vi "SCA-RT.vi"() -> ()   [LabVIEW 2016]
uses:
  controls/SCA states.ctl
  Common-Control/Gate Valve Readback.ctl
  controls/Vertical Rod states.ctl
  Common-Control/Horizontal Rod states.ctl
  Common-Control/GP307 cluster.ctl
  controls/SCA commands.ctl
  controls/SCA Bypass control.ctl
  <vilib>/Platform/TimedLoop/XDataNode/timing_clust.ctl
  <vilib>/Platform/TimedLoop/XDataNode/nitl_modes.ctl
  <vilib>/Platform/TimedLoop/XDataNode/wakeup.ctl
  controls/Encoder bit cluster.ctl
  controls/Minimum Times.ctl
  <vilib>/Analysis/baseanly.llb/Mean (DBL).vi
  <vilib>/Instr/_visa.llb/VISA Configure Serial Port (Instr).vi
  <vilib>/Motion/Express/_s/nimc.fb.straightLineMove.startStraightLineMove.axis.modeRelative.0.vi
  <vilib>/Platform/TimedLoop/XDataNode/loadnilvce.vi
  <vilib>/Motion/BlockNode/FB.NIMotion.xnode
  <vilib>/Platform/TimedLoop/XDataNode/XDataNode.xnode
  <vilib>/Platform/TimedLoop/XDataNode/XDNodeRunTimeDep.lvlib
  <vilib>/Analysis/NI_AALBase.lvlib
  <vilib>/NI_Real-Time Target Support.lvlib
panel:
  in  "Insert Rod Bypass":bool
  in  "Retract Rod Bypass":bool
  in  "Sample Rod Bypass":bool
  in  "Wheel GV Bypass":bool
  out "Bypass Control":T1
  out "Timeouts":T2
  out "Immersion Lens I set":dbl
  out "Immersion Lens V Set":dbl
  out "Timeouts Update loop error":errorcluster
  out "SCA Command":T3
  out "Encoder loop error":errorcluster
  out "Convectron readback loop error":errorcluster
  out "HV Control loop error":errorcluster
  out "Rotate Wheel error":errorcluster
  out "Ion Source Vac Cluster":T4
  out "Bellows Vac Cluster":T4
  out "SCA-cRIO error":errorcluster
  in  "Rollover Sample":i8=54
  out "Insert Rod Status":T5
  out "Retract Rod Status":T5
  out "Sample Rod status":T6
  out "Wheel GV":T7
  out "Raw bits":bool[](array[boolean])
  out "Converted bits":bool[](array[boolean])
  out "Immersion Lens I read":dbl format="%0.2f"
  out "Immersion Lens V read":dbl format="%0.2f"
  out "SCA next state":T8
  out "Extractor I read":dbl
  out "Extractor V read":dbl
  out "Extractor V set":dbl
  out "Cathode V read":dbl
  out "Cathode I read":dbl
  out "Cathode V set":dbl
  out "New Move":dbl
  out "Encoder Destination":dbl
  in  "Step Window Radius":i16=2
  out "In Range?":bool
  out "Window Limit 2":u32
  out "Window Limit 1":u32
  out "Encoder position":u16
  in  "clear error 3":bool
  in  "clear error 2":bool
  in  "clear error":bool
  out "action":string
  out "Vac Readback Loop error":errorcluster
  out "Sample Wheel Convectron":string
  out "Sample Rod UP sensor":bool
  out "Sample Rod DOWN sensor":bool
  out "Rotation done":bool
  out "Insert Rod IN sensor":bool
  out "Insert Rod OUT sensor":bool
  out "Retract Rod IN sensor":bool
  out "Retract Rod OUT sensor":bool
  out "Sensor loop error":errorcluster
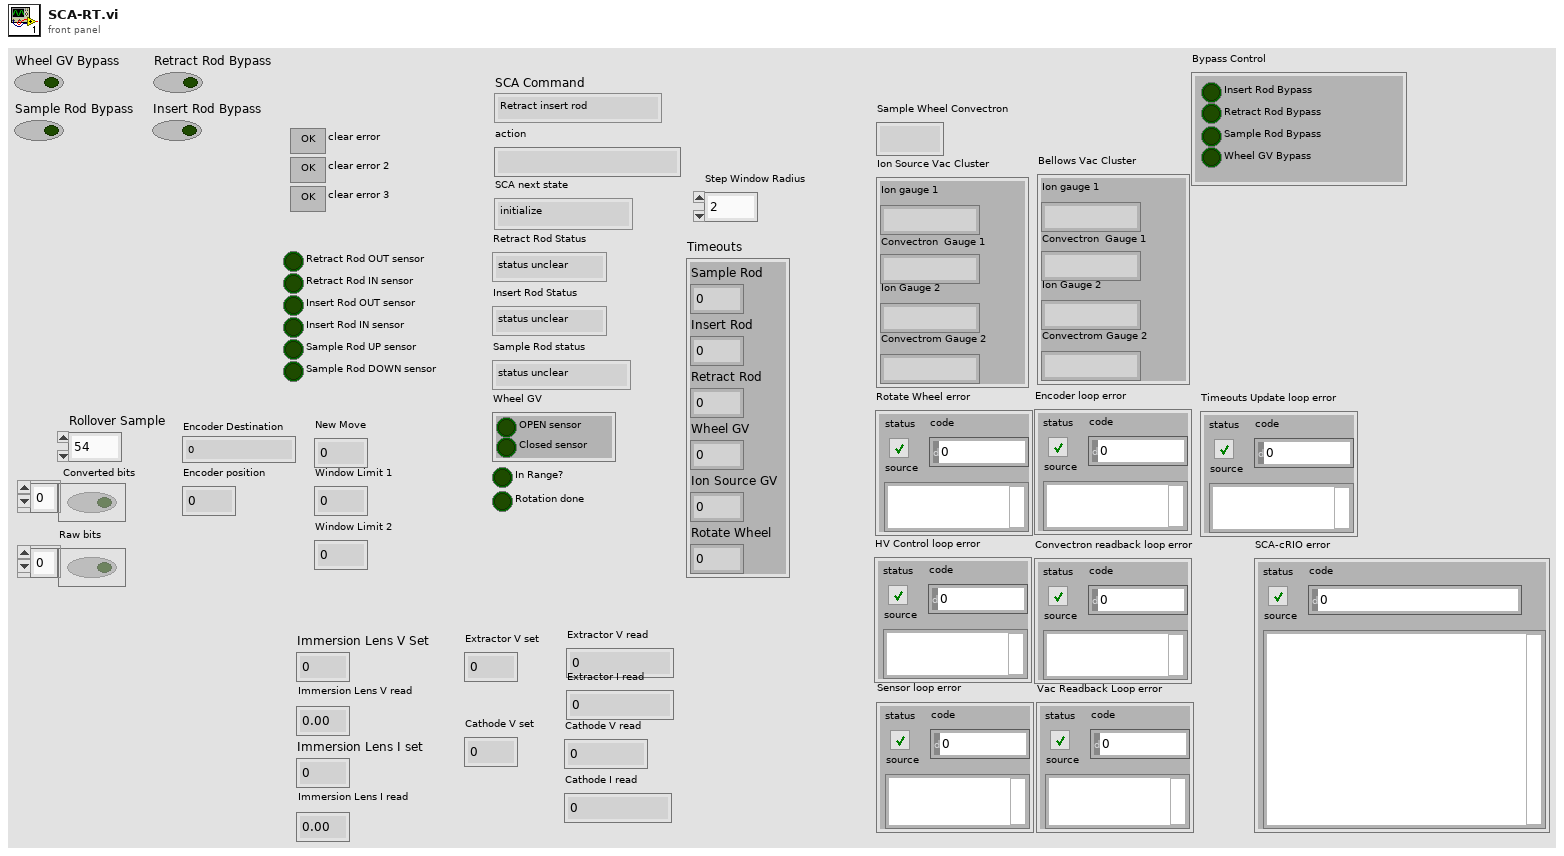
[diagram p1: front panel]
types:
  T1 = typedef "SCA Bypass control.ctl" = cluster{"Insert Rod Bypass":bool, "Retract Rod Bypass":bool, "Sample Rod Bypass":bool, "Wheel GV Bypass":bool}
  T2 = cluster{"Sample Rod":u16, "Insert Rod":u16, "Retract Rod":u16, "Wheel GV":u16, "Ion Source GV":u16, "Rotate Wheel":u16}
  T3 = typedef "SCA commands.ctl" = enum16{"Retract insert rod", "Insert insert rod", "Retract retract rod", "Insert retract rod", "Retract sample rod", "Insert sample rod", "Open wheel GV", "Close wheel GV", "Open ion source GV", "Close ion source GV", "Pump out source", "Vent source", "Rotate wheel randomly", "Rotate wheel", "Start random sample change", "Start sample change"}
  T4 = typedef "GP307 cluster.ctl" = cluster{"Ion gauge 1":string, "Convectron  Gauge 1 ":string, "Ion Gauge 2":string, "Convectrom Gauge 2":string}
  T5 = typedef "Horizontal Rod states.ctl" = enum16{"status unclear", "rod in", "rod out"}
  T6 = typedef "Vertical Rod states.ctl" = enum16{"status unclear", "rod down", "rod up"}
  T7 = typedef "Gate Valve Readback.ctl" = cluster{"OPEN sensor":bool, "Closed sensor":bool}
  T8 = typedef "SCA states.ctl" = enum16{"initialize", "wait", "change sample start", "change sample", "check position", "rotate wheel", "sample change complete", "sample rod up", "sample rod down", "retract rod in", "retract rod out", "insert rod in", "insert rod out", "wheel GV open", "wheel GV close", "vent source", "pump source"}
  T9 = cluster{"Sample Rod":u32, "Insert Rod":u32, "Retract Rod":u32, "Wheel GV":u32, "Ion Source GV":u32, "Rotate Wheel":u32}
  T10 = typedef "Minimum Times.ctl" = cluster{"Rotate Wheel Minimum Time":u32}
  T11 = typedef "GV states.ctl" = enum16{"status unclear", "closed", "open"}
  T12 = typedef "XDNodeRunTimeDep.lvlib/timing_clust.ctl" = cluster{"Expected End [f-1]":u64, "Actual End [f-1]":u64, "Finished Late? [f-1]":bool, "Expected End [i-1]":u64, "Actual End [i-1]":u64, "Finished Late? [i-1]":bool, "Expected Start [i]":u64, "Actual Start [i]":u64, "Expected Start [f]":u64, "Actual Start [f]":u64, "Source Name":string, "Structure Name":string, "Period":i64, "Deadline":i64, "Offset":i64, "Start":i64, "Priority":i32, "Timeout":i32, "Mode":T13, "Wakeup Reason":T14, "Error":errorcluster, "Source Type":string, "Secondary Source Type":string, "Global End Time":u64, "Global Start Time":u64, "Frame Duration":u64, "Iteration Duration":u64, "Assigned CPU":i32, "I/O Scan Engine Mode":u32}
  T13 = typedef "XDNodeRunTimeDep.lvlib/nitl_modes.ctl" = enum32{"No Change", "Process missed periods, maintain original phase", "Discard missed periods, maintain original phase", "Process missed periods, ignore original phase", "Discard missed periods, ignore original phase"}
  T14 = typedef "XDNodeRunTimeDep.lvlib/wakeup.ctl" = enum32{"Normal", "Aborted", "Asynchronous wakeup", "Timing source error", "Timed loop error", "Timeout"}
  T15 = typedef "Encoder bit cluster.ctl" = cluster{"MSB":bool, "13th bit":bool, "12th bit":bool, "11th bit":bool, "10th bit":bool, "9th bit":bool, "8th bit":bool, "7th bit":bool, "6th bit":bool, "5th bit":bool, "4th bit":bool, "3rd bit":bool, "2nd bit":bool, "LSB":bool}
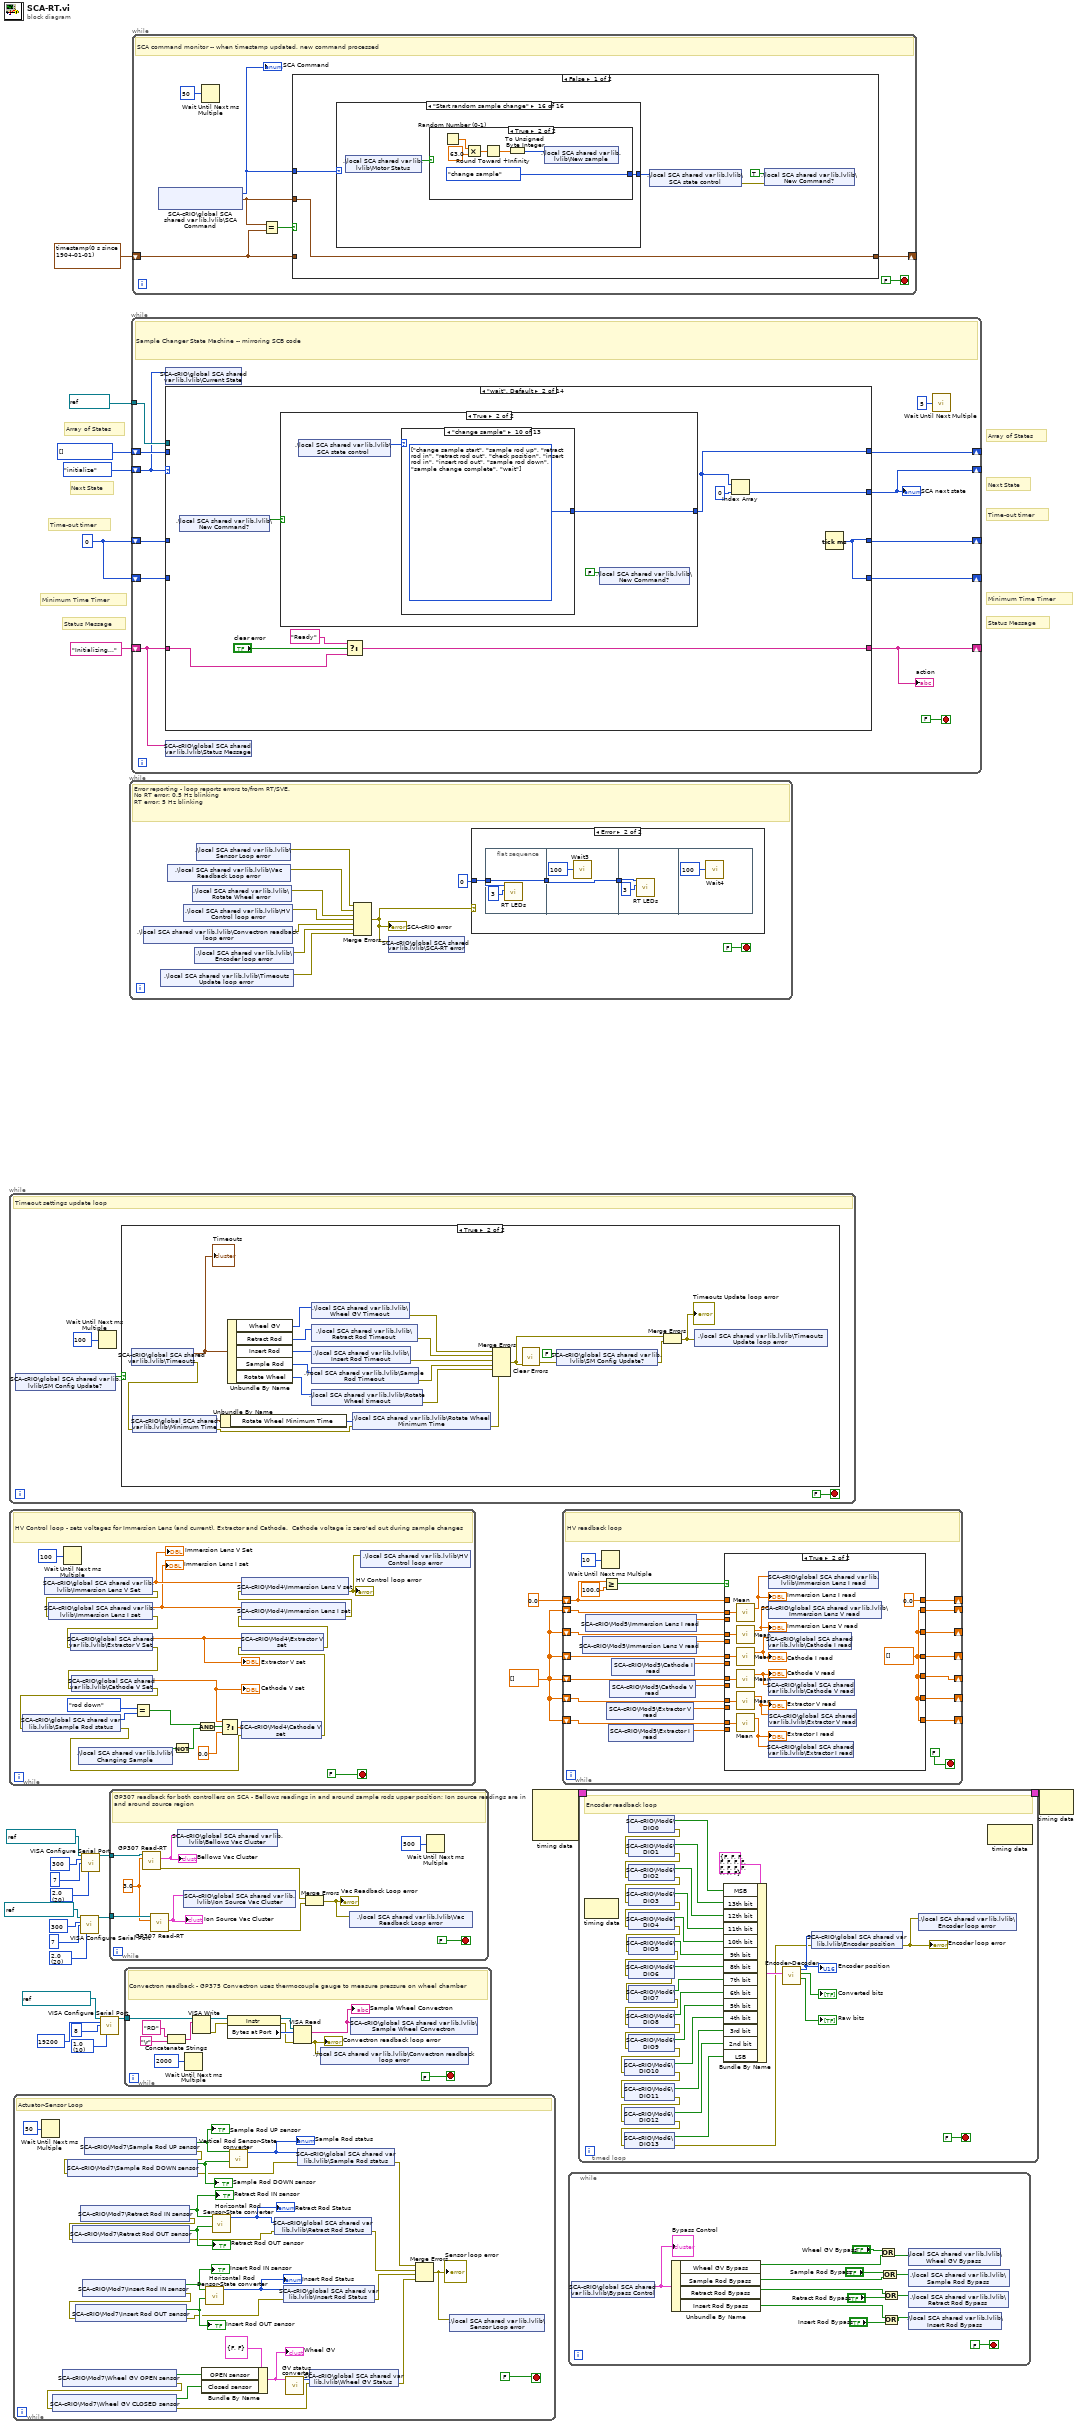
[diagram p0: block diagram]
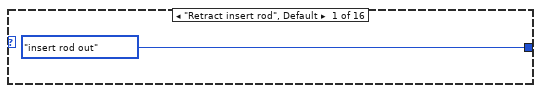
[diagram p2: hidden frame]
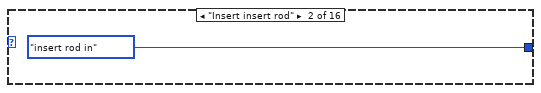
[diagram p3: hidden frame]
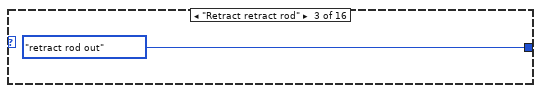
[diagram p4: hidden frame]
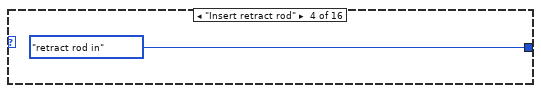
[diagram p5: hidden frame]
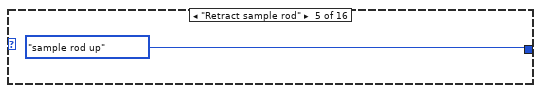
[diagram p6: hidden frame]
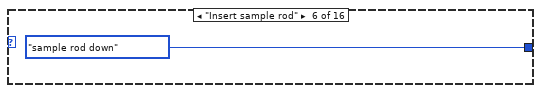
[diagram p7: hidden frame]
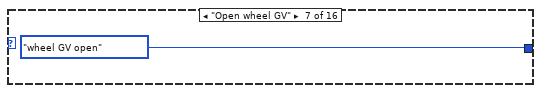
[diagram p8: hidden frame]
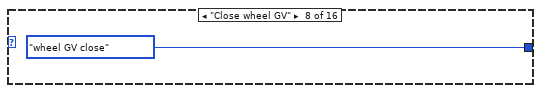
[diagram p9: hidden frame]
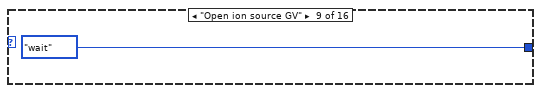
[diagram p10: hidden frame]
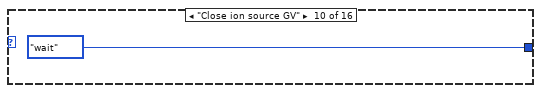
[diagram p11: hidden frame]
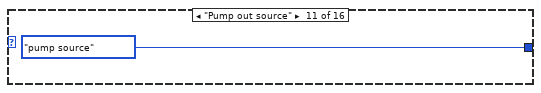
[diagram p12: hidden frame]
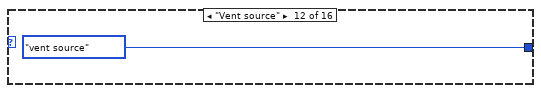
[diagram p13: hidden frame]
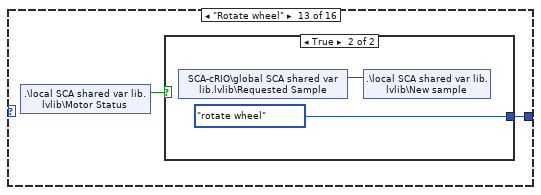
[diagram p14: hidden frame]
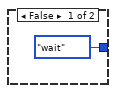
[diagram p15: hidden frame]
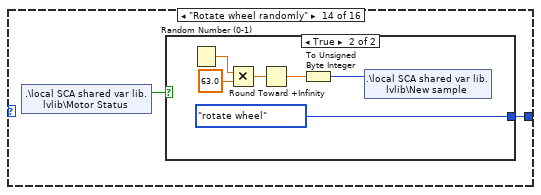
[diagram p16: hidden frame]
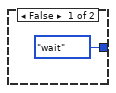
[diagram p17: hidden frame]
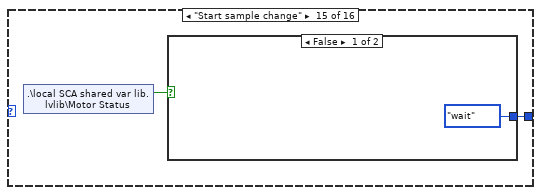
[diagram p18: hidden frame]
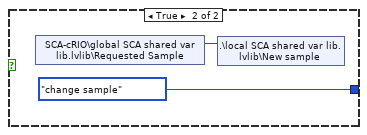
[diagram p19: hidden frame]
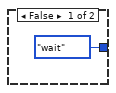
[diagram p20: hidden frame]
diagram:
  w3 = dbl[] []
  w20 = u16 20 items=["1.0"=10, "1.5"=15, "2.0"=20] ("stop bits (10: 1 bit)")
  w24 = u16 10 items=["1.0"=10, "1.5"=15, "2.0"=20] ("stop bits (10: 1 bit)")
  w14 = u16 20 items=["1.0"=10, "1.5"=15, "2.0"=20] ("stop bits (10: 1 bit)")
  w8 = u32 0
  w25 = T8[] [] items=["initialize", "wait", "change sample start", "change sample", "check position", "rotate wheel", "sample change complete", "sample rod up", "sample rod down", "retract rod in", "retract rod out", "insert rod in", "insert rod out", "wheel GV open", "wheel GV close", "vent source", "pump source"]
  # "Status Message"
  # "Array of States"
  # "Next State"
  # "Time-out timer"
  # "Minimum Time Timer"
  # "Status Message"
  # "Array of States"
  # "Next State"
  # "Time-out timer"
  # "Minimum Time Timer"
  n1 = while {
    stop <- FALSE stop-if-true
    # "Timeout settings update loop"
    n2 = shared-variable "SCA-cRIO\\global SCA shared var lib.lvlib\\SM Config Update?"() -> (w28:bool)  [unwired: 1 in, 1 out]
    n3 = Wait Until Next ms Multiple(millisecond multiple=u32 100) -> ()  [unwired: 1 out]
    n4 = case shown="True" w28 {
      frame False {
      }
      frame True {
        n5 = shared-variable "SCA-cRIO\\global SCA shared var lib.lvlib\\Timeouts"() -> (w48:T9, error out=w31:errorcluster)  [unwired: 1 in]
        "Timeouts" <- w48
        n6 = shared-variable "SCA-cRIO\\global SCA shared var lib.lvlib\\Minimum Time"(error in=w31) -> (w33:T10, error out=w30:errorcluster)
        n7 = Unbundle By Name(w33) -> ("Rotate Wheel Minimum Time"=w32:u32)
        n8 = Unbundle By Name(w48) -> ("Wheel GV"=w47:u32, "Retract Rod"=w34:u32, "Insert Rod"=w41:u32, "Sample Rod"=w38:u32, "Rotate Wheel"=w37:u32)
        n9 = shared-variable ".\\local SCA shared var lib.lvlib\\Wheel GV Timeout"(w47) -> (error out=w46:errorcluster)  [unwired: 1 in]
        n10 = shared-variable ".\\local SCA shared var lib.lvlib\\Retract Rod Timeout"(w34) -> (error out=w40:errorcluster)  [unwired: 1 in]
        n11 = shared-variable ".\\local SCA shared var lib.lvlib\\Insert Rod Timeout"(w41) -> (error out=w39:errorcluster)  [unwired: 1 in]
        n12 = shared-variable ".\\local SCA shared var lib.lvlib\\Sample Rod Timeout"(w38) -> (error out=w36:errorcluster)  [unwired: 1 in]
        n13 = shared-variable ".\\local SCA shared var lib.lvlib\\Rotate Wheel timeout"(w37) -> (error out=w35:errorcluster)  [unwired: 1 in]
        n14 = shared-variable ".\\local SCA shared var lib.lvlib\\Rotate Wheel Minimum Time"(w32, error in=w30) -> (error out=w29:errorcluster)
        n15 = Merge Errors(w46, w40, w39, w36, w35, w29) -> (w44:errorcluster)
        n16 = call <vilib>:"Clear Errors.vi"("error in (no error)"=w44) -> ("error out"=w45:errorcluster)  [unwired: 5 in, 1 out]
        n17 = shared-variable "SCA-cRIO\\global SCA shared var lib.lvlib\\SM Config Update?"(FALSE ("SM Config Update?"), error in=w45) -> (error out=w43:errorcluster)
        n18 = Merge Errors(w44, w43) -> (w42:errorcluster)
        "Timeouts Update loop error" <- w42
        n19 = shared-variable ".\\local SCA shared var lib.lvlib\\Timeouts Update loop error"(w42) -> ()  [unwired: 1 in, 1 out]
      }
    }
  }
  n20 = while {
    stop <- FALSE stop-if-true
    # "HV Control loop - sets voltages for Immersion Lens (and current), Extractor and Cathode.  Cathode voltage is zero'ed out during sample changes"
    n21 = shared-variable "SCA-cRIO\\global SCA shared var lib.lvlib\\Immersion Lens V Set"() -> (w64:dbl, error out=w62:errorcluster)  [unwired: 1 in]
    "Immersion Lens V Set" <- w64
    n22 = shared-variable "SCA-cRIO\\global SCA shared var lib.lvlib\\Immersion Lens I set"(error in=w62) -> (w63:dbl, error out=w61:errorcluster)
    "Immersion Lens I set" <- w63
    n23 = Wait Until Next ms Multiple(millisecond multiple=u32 100) -> ()  [unwired: 1 out]
    n24 = shared-variable "SCA-cRIO\\global SCA shared var lib.lvlib\\Extractor V Set"(error in=w61) -> (w70:dbl, error out=w60:errorcluster)
    "Extractor V set" <- w70
    n25 = shared-variable "SCA-cRIO\\global SCA shared var lib.lvlib\\Cathode V Set"(error in=w60) -> (w67:dbl, error out=w59:errorcluster)
    "Cathode V set" <- w67
    n26 = shared-variable "SCA-cRIO\\global SCA shared var lib.lvlib\\Sample Rod status"(error in=w59) -> (w53:T6, error out=w51:errorcluster)
    n27 = shared-variable ".\\local SCA shared var lib.lvlib\\Changing Sample"() -> (w69:bool)  [unwired: 1 in, 1 out]
    n28 = Equal?(x=Vertical_Rod_states."rod down", y=w53) -> (x = y?=w54:bool)
    n29 = Not(x=w69) -> (.not. x?=w50:bool)
    n30 = And(x=w54, y=w50) -> (x .and. y?=w68:bool)
    n31 = Select(t=w67, s=w68, f=0.0) -> (s? t:f=w65:dbl)
    n32 = shared-variable "SCA-cRIO\\Mod4\\Cathode V set"(w65, error in=w51) -> (error out=w56:errorcluster)
    n33 = shared-variable "SCA-cRIO\\Mod4\\Extractor V set"(w70, error in=w56) -> (error out=w57:errorcluster)
    n34 = shared-variable "SCA-cRIO\\Mod4\\Immersion Lens I set"(w63, error in=w57) -> (error out=w58:errorcluster)
    n35 = shared-variable "SCA-cRIO\\Mod4\\Immersion Lens V set"(w64, error in=w58) -> (error out=w55:errorcluster)
    "HV Control loop error" <- w55
    n36 = shared-variable ".\\local SCA shared var lib.lvlib\\HV Control loop error"(w55) -> ()  [unwired: 1 in, 1 out]
  }
  n37 = while {
    stop <- FALSE ("stop") stop-if-true
    # "Actuator-Sensor Loop"
    n38 = Wait Until Next ms Multiple(millisecond multiple=u32 50) -> ()  [unwired: 1 out]
    n39 = shared-variable "SCA-cRIO\\Mod7\\Wheel GV OPEN sensor"() -> (w96:bool, error out=w82:errorcluster)  [unwired: 1 in]
    n40 = shared-variable "SCA-cRIO\\Mod7\\Wheel GV CLOSED sensor"(error in=w82) -> (w97:bool, error out=w81:errorcluster)
    n41 = shared-variable "SCA-cRIO\\Mod7\\Retract Rod IN sensor"() -> (w91:bool, error out=w84:errorcluster)  [unwired: 1 in]
    "Retract Rod IN sensor" <- w91
    n42 = shared-variable "SCA-cRIO\\Mod7\\Retract Rod OUT sensor"(error in=w84) -> (w90:bool, error out=w78:errorcluster)
    "Retract Rod OUT sensor" <- w90
    n43 = shared-variable "SCA-cRIO\\Mod7\\Insert Rod IN sensor"() -> (w89:bool, error out=w83:errorcluster)  [unwired: 1 in]
    "Insert Rod IN sensor" <- w89
    n44 = shared-variable "SCA-cRIO\\Mod7\\Insert Rod OUT sensor"(error in=w83) -> (w88:bool, error out=w80:errorcluster)
    "Insert Rod OUT sensor" <- w88
    n45 = shared-variable "SCA-cRIO\\Mod7\\Sample Rod UP sensor"() -> (w94:bool, error out=w85:errorcluster)  [unwired: 1 in]
    "Sample Rod UP sensor" <- w94
    n46 = shared-variable "SCA-cRIO\\Mod7\\Sample Rod DOWN sensor"(error in=w85) -> (w93:bool, error out=w79:errorcluster)
    "Sample Rod DOWN sensor" <- w93
    n47 = Bundle By Name(cluster=T7 {"OPEN sensor"=FALSE, "Closed sensor"=FALSE} ("Gate Valve"), "OPEN sensor"=w96, "Closed sensor"=w97) -> (w99:T7)
    "Wheel GV" <- w99
    n48 = call "Horizontal Rod Sensor-State converter.vi"("IN Sensor"=w89, "OUT Sensor"=w88) -> ("Status"=w87:T5)  [unwired: 8 in]
    "Insert Rod Status" <- w87
    n49 = call "Horizontal Rod Sensor-State converter.vi"("IN Sensor"=w91, "OUT Sensor"=w90) -> ("Status"=w86:T5)  [unwired: 8 in]
    "Retract Rod Status" <- w86
    n50 = call "Vertical Rod Sensor-State converter.vi"("UP Sensor"=w94, "DOWN Sensor"=w93) -> ("Status"=w92:T6)  [unwired: 8 in]
    "Sample Rod status" <- w92
    n51 = shared-variable "SCA-cRIO\\global SCA shared var lib.lvlib\\Retract Rod Status"(w86, error in=w78) -> (error out=w75:errorcluster)
    n52 = shared-variable "SCA-cRIO\\global SCA shared var lib.lvlib\\Insert Rod Status"(w87, error in=w80) -> (error out=w74:errorcluster)
    n53 = call "GV status converter.vi"("Gate Valve"=w99) -> ("GV Status"=w95:T11)  [unwired: 10 in]
    n54 = shared-variable "SCA-cRIO\\global SCA shared var lib.lvlib\\Sample Rod status"(w92, error in=w79) -> (error out=w76:errorcluster)
    n55 = shared-variable "SCA-cRIO\\global SCA shared var lib.lvlib\\Wheel GV Status"(w95, error in=w81) -> (error out=w73:errorcluster)
    n56 = Merge Errors(w76, w75, w74, w73) -> (w77:errorcluster)
    "Sensor loop error" <- w77
    n57 = shared-variable ".\\local SCA shared var lib.lvlib\\Sensor Loop error"(w77) -> ()  [unwired: 1 in, 1 out]
  }
  n58 = call-poly "VISA Configure Serial Port"("VISA resource name"=refnum<visa-resource-name> "ASRL6::INSTR", "baud rate (9600)"=u32 300, "data bits (8)"=u16 7, "stop bits (10: 1 bit)"=w14) -> ("VISA resource name out"=w15:refnum<visa-resource-name>)  [unwired: 10 in, 1 out]
  n59 = call-poly "VISA Configure Serial Port"("VISA resource name"=refnum<visa-resource-name> "ASRL8::INSTR", "baud rate (9600)"=u32 300, "data bits (8)"=u16 7, "stop bits (10: 1 bit)"=w20) -> ("VISA resource name out"=w21:refnum<visa-resource-name>)  [unwired: 10 in, 1 out]
  n60 = call-poly "VISA Configure Serial Port"("VISA resource name"=refnum<visa-resource-name> "ASRL7::INSTR", "baud rate (9600)"=u32 19200, "data bits (8)"=u16 8, "stop bits (10: 1 bit)"=w24) -> ("VISA resource name out"=w10:refnum<visa-resource-name>)  [unwired: 10 in, 1 out]
  n61 = while {
    tunnel: w15 -> [w105]
    tunnel: w21 -> [w108]
    stop <- FALSE ("stop 4") stop-if-true
    w104 = 3.0 ("Delay Time (s)")
    # "GP307 readback for both controllers on SCA - Bellows readings in and around sample rods upper position; Ion source readings are in and around source region"
    n62 = call "GP307 Read-RT.vi"("Delay Time (s)"=w104, "VISA Refnum in"=w108) -> ("error out"=w106:errorcluster, "GP307 output"=w107:T4)  [unwired: 7 in, 1 out]
    "Bellows Vac Cluster" <- w107
    n63 = call "GP307 Read-RT.vi"("Delay Time (s)"=w104, "VISA Refnum in"=w105) -> ("error out"=w102:errorcluster, "GP307 output"=w103:T4)  [unwired: 7 in, 1 out]
    "Ion Source Vac Cluster" <- w103
    n64 = shared-variable "SCA-cRIO\\global SCA shared var lib.lvlib\\Bellows Vac Cluster"(w107) -> ()  [unwired: 1 in, 1 out]
    n65 = shared-variable "SCA-cRIO\\global SCA shared var lib.lvlib\\Ion Source Vac Cluster"(w103) -> ()  [unwired: 1 in, 1 out]
    n66 = Merge Errors(w106, w102) -> (w109:errorcluster)
    "Vac Readback Loop error" <- w109
    n67 = shared-variable ".\\local SCA shared var lib.lvlib\\Vac Readback Loop error"(w109) -> ()  [unwired: 1 in, 1 out]
    n68 = Wait Until Next ms Multiple(millisecond multiple=u32 500) -> ()  [unwired: 1 out]
  }
  n69 = while {
    tunnel: w10 -> [w117]
    stop <- FALSE ("stop 3") stop-if-true
    # "Convectron readback - GP375 Convectron uses thermocouple gauge to measure pressure on wheel chamber"
    n70 = Concatenate Strings("RD" ("write buffer 2"), "\r") -> (w124:string)
    n71 = Wait Until Next ms Multiple(millisecond multiple=u32 2000) -> ()  [unwired: 1 out]
    n72 = VISA Write(VISA resource name=w117, write buffer=w124) -> (VISA resource name out=w118:refnum<visa-resource-name>, error out=w114:errorcluster)  [unwired: 1 in, 1 out]
    n73 = property class="Instr"(reference=w118, error in=w114) -> (reference out=w119:refnum<visa-resource-name>, error out=w113:errorcluster, "Bytes at Port"=w120:u32)
    n74 = VISA Read(VISA resource name=w119, byte count=w120, error in (no error)=w113) -> (read buffer=w115:string, error out=w112:errorcluster)  [unwired: 2 out]
    "Sample Wheel Convectron" <- w115
    "Convectron readback loop error" <- w112
    n75 = shared-variable ".\\local SCA shared var lib.lvlib\\Convectron readback loop error"(w112) -> ()  [unwired: 1 in, 1 out]
    n76 = shared-variable "SCA-cRIO\\global SCA shared var lib.lvlib\\Sample Wheel Convectron"(w115) -> ()  [unwired: 1 in, 1 out]
  }
  n77 = while {
    stop <- FALSE stop-if-true
    # "Error reporting - loop reports errors to/from RT/SVE. \nNo RT error: 0.5 Hz blinking\nRT error: 5 Hz blinking"
    n78 = shared-variable ".\\local SCA shared var lib.lvlib\\Convectron readback loop error"() -> (w127:errorcluster)  [unwired: 1 in, 1 out]
    n79 = shared-variable ".\\local SCA shared var lib.lvlib\\Timeouts Update loop error"() -> (w125:errorcluster)  [unwired: 1 in, 1 out]
    n80 = shared-variable ".\\local SCA shared var lib.lvlib\\Vac Readback Loop error"() -> (w132:errorcluster)  [unwired: 1 in, 1 out]
    n81 = shared-variable ".\\local SCA shared var lib.lvlib\\HV Control loop error"() -> (w128:errorcluster)  [unwired: 1 in, 1 out]
    n82 = shared-variable ".\\local SCA shared var lib.lvlib\\Rotate Wheel error"() -> (w129:errorcluster)  [unwired: 1 in, 1 out]
    n83 = shared-variable ".\\local SCA shared var lib.lvlib\\Encoder loop error"() -> (w126:errorcluster)  [unwired: 1 in, 1 out]
    n84 = shared-variable ".\\local SCA shared var lib.lvlib\\Sensor Loop error"() -> (w133:errorcluster)  [unwired: 1 in, 1 out]
    n85 = Merge Errors(w133, w132, w129, w128, w127, w126, w125) -> (w131:errorcluster)
    "SCA-cRIO error" <- w131
    n86 = shared-variable "SCA-cRIO\\global SCA shared var lib.lvlib\\SCA-RT error"(w131) -> ()  [unwired: 1 in, 1 out]
    n87 = case shown="Error" w131 {
      tunnel: 0 -> [w137 w145]
      frame No Error {
        n88 = flat-sequence {
          tunnel: w137 -> [w138]
          tunnel: [w138] -> w135
          tunnel: [w140] -> w136
          tunnel: w135 -> [w140]
          tunnel: w136 -> [w142]
          frame #0 {
            n89 = call <vilib>:"RT LEDs.vi"("State"=3, "LED Num"=w138) -> ()  [unwired: 4 in, 2 out]
          }
          frame #1 {
            n90 = call "Wait"("Count(mSec)"=u16 1000) -> ()  [unwired: 1 out]
          }
          frame #2 {
            n91 = call <vilib>:"RT LEDs.vi"("State"=3, "LED Num"=w142) -> ()  [unwired: 4 in, 2 out]
          }
          frame #3 {
            n92 = call "Wait2"("Count(mSec)"=u16 1000) -> ()  [unwired: 1 out]
          }
        }
      }
      frame Error {
        n93 = flat-sequence {
          tunnel: [w148] -> w147
          tunnel: w145 -> [w148]
          tunnel: w147 -> [w150]
          tunnel: [w150] -> w146
          tunnel: w146 -> [w152]
          frame #0 {
            n94 = call <vilib>:"RT LEDs.vi"("State"=3, "LED Num"=w148) -> ()  [unwired: 4 in, 2 out]
          }
          frame #1 {
            n95 = call "Wait3"("Count(mSec)"=u16 100) -> ()  [unwired: 1 out]
          }
          frame #2 {
            n96 = call <vilib>:"RT LEDs.vi"("State"=3, "LED Num"=w152) -> ()  [unwired: 4 in, 2 out]
          }
          frame #3 {
            n97 = call "Wait4"("Count(mSec)"=u16 100) -> ()  [unwired: 1 out]
          }
        }
      }
    }
  }
  n98 = while {
    shift-right: [w155] -> _
    shift-left: SCA_states."initialize" ("SC2 state") -> [w156]
    shift-right: [w159] -> _
    shift-left: w25 -> [w165]
    shift-right: [w163] -> _
    shift-left: w8 -> [w164]
    shift-right: [w157] -> _
    shift-left: "Initializing..." -> [w160]
    shift-right: [w161] -> _
    shift-left: w8 -> [w162]
    tunnel: refnum<k21> "Axis 1" ("resource") -> [w166]
    stop <- FALSE ("stop 2") stop-if-true
    # "Sample Changer State Machine -- mirroring SCB code"
    n99 = shared-variable "SCA-cRIO\\global SCA shared var lib.lvlib\\Current State"(w156) -> ()  [unwired: 1 in, 1 out]
    n100 = case shown="\"wait\", Default" w156 {
      selector: w156 -> [_ _ w208 w241 w305 w333 w402 w468 w496 w569 w592 _ w659 w740]
      tunnel: w166 -> [_ _ _ _ _ _ _ _ _ _ _ w615 w655 _]
      tunnel: [SCA_states."wait" ("SC2 state") w184 w213 w237 w300 w328 w397 w463 w491 w565 w590 w603 w656 w738] -> w155
      tunnel: w165 -> [w176 _ w210 w243 w306 w334 w403 w469 w497 w570 w594 w604 w654 w741]
      tunnel: w164 -> [w179 _ w209 w239 w303 w330 w400 w466 w493 w567 _ w607 w651 _]
      tunnel: [w179 w183 w209 w239 w303 w330 w400 w466 w493 w567 w595 w607 w657 w744] -> w163
      tunnel: [w176 w185 w212 w236 w299 w327 w396 w462 w492 w564 w593 w604 w653 w739] -> w159
      tunnel: w160 -> [w177 w189 _ _ _ _ _ _ _ _ w598 _ _ w748]
      tunnel: [w177 w188 w214 w240 w302 w331 w399 w465 w494 w563 w591 "done rotating, checking position" ("t") w652 w747] -> w157
      tunnel: w162 -> [w180 _ w215 w242 w304 w332 w401 w467 w495 w568 _ w606 w648 _]
      tunnel: [w180 w183 w211 w238 w301 w329 w398 w464 w490 w566 w595 w606 w658 w744] -> w161
      frame "initialize" {
        n101 = shared-variable ".\\local SCA shared var lib.lvlib\\Motor Status"(TRUE ("Motor Status")) -> ()  [unwired: 1 in, 1 out]
        n102 = shared-variable ".\\local SCA shared var lib.lvlib\\Changing Sample"(FALSE ("Changing Sample")) -> ()  [unwired: 1 in, 1 out]
        n103 = shared-variable "SCA-cRIO\\global SCA shared var lib - old.lvlib\\Start Sample Change"(FALSE ("start sample change")) -> ()  [unwired: 1 in, 1 out]
        n104 = shared-variable ".\\local SCA shared var lib.lvlib\\Rotate Wheel Minimum Time"(u16 1000 ("Rotate Wheel Minimum Time")) -> ()  [unwired: 1 in, 1 out]
        n105 = shared-variable ".\\local SCA shared var lib.lvlib\\Retract Rod Timeout"(u32 10000 ("Retract Rod Timeout")) -> ()  [unwired: 1 in, 1 out]
        n106 = shared-variable ".\\local SCA shared var lib.lvlib\\Wheel GV Timeout"(10000 ("Wheel GV Timeout")) -> ()  [unwired: 1 in, 1 out]
        n107 = shared-variable ".\\local SCA shared var lib.lvlib\\Rotate Wheel timeout"(u32 30000 ("Rotate Wheel timeout")) -> ()  [unwired: 1 in, 1 out]
        n108 = shared-variable ".\\local SCA shared var lib.lvlib\\Sample Rod Timeout"(u32 10000 ("Sample Rod Timeout")) -> ()  [unwired: 1 in, 1 out]
        n109 = shared-variable ".\\local SCA shared var lib.lvlib\\Insert Rod Timeout"(u32 10000 ("Insert Rod Timeout")) -> ()  [unwired: 1 in, 1 out]
      }
      frame "wait", Default {
        n110 = shared-variable ".\\local SCA shared var lib.lvlib\\New Command?"() -> (w182:bool)  [unwired: 1 in, 1 out]
        n111 = case shown="True" w182 {
          tunnel: [w191 w194] -> w185
          frame False {
            w191 = T8[] [enum."wait"] items=["initialize", "wait", "change sample start", "change sample", "check position", "rotate wheel", "sample change complete", "sample rod up", "sample rod down", "retract rod in", "retract rod out", "insert rod in", "insert rod out", "wheel GV open", "wheel GV close", "vent source", "pump source"]
          }
          frame True {
            n112 = shared-variable ".\\local SCA shared var lib.lvlib\\SCA state control"() -> (w193:T8)  [unwired: 1 in, 1 out]
            n113 = case shown="\"change sample\"" w193 {
              tunnel: [w195 w196 w197 w198 w199 w200 w201 w202 w203 w204 w205 w206 w207] -> w194
              frame "wheel GV close" {
                w195 = T8[] [enum."wheel GV close", enum."wait"] items=["initialize", "wait", "change sample start", "change sample", "check position", "rotate wheel", "sample change complete", "sample rod up", "sample rod down", "retract rod in", "retract rod out", "insert rod in", "insert rod out", "wheel GV open", "wheel GV close", "vent source", "pump source"]
              }
              frame "wheel GV open" {
                w196 = T8[] [enum."wheel GV open", enum."wait"] items=["initialize", "wait", "change sample start", "change sample", "check position", "rotate wheel", "sample change complete", "sample rod up", "sample rod down", "retract rod in", "retract rod out", "insert rod in", "insert rod out", "wheel GV open", "wheel GV close", "vent source", "pump source"]
              }
              frame "sample rod up" {
                w197 = T8[] [enum."sample rod up", enum."wait"] items=["initialize", "wait", "change sample start", "change sample", "check position", "rotate wheel", "sample change complete", "sample rod up", "sample rod down", "retract rod in", "retract rod out", "insert rod in", "insert rod out", "wheel GV open", "wheel GV close", "vent source", "pump source"]
              }
              frame "sample rod down" {
                w198 = T8[] [enum."sample rod down", enum."wait"] items=["initialize", "wait", "change sample start", "change sample", "check position", "rotate wheel", "sample change complete", "sample rod up", "sample rod down", "retract rod in", "retract rod out", "insert rod in", "insert rod out", "wheel GV open", "wheel GV close", "vent source", "pump source"]
              }
              frame "retract rod in" {
                w199 = T8[] [enum."retract rod in", enum."wait"] items=["initialize", "wait", "change sample start", "change sample", "check position", "rotate wheel", "sample change complete", "sample rod up", "sample rod down", "retract rod in", "retract rod out", "insert rod in", "insert rod out", "wheel GV open", "wheel GV close", "vent source", "pump source"]
              }
              frame "retract rod out" {
                w200 = T8[] [enum."retract rod out", enum."wait"] items=["initialize", "wait", "change sample start", "change sample", "check position", "rotate wheel", "sample change complete", "sample rod up", "sample rod down", "retract rod in", "retract rod out", "insert rod in", "insert rod out", "wheel GV open", "wheel GV close", "vent source", "pump source"]
              }
              frame "insert rod in" {
                w201 = T8[] [enum."insert rod in", enum."wait"] items=["initialize", "wait", "change sample start", "change sample", "check position", "rotate wheel", "sample change complete", "sample rod up", "sample rod down", "retract rod in", "retract rod out", "insert rod in", "insert rod out", "wheel GV open", "wheel GV close", "vent source", "pump source"]
              }
              frame "insert rod out" {
                w202 = T8[] [enum."insert rod out", enum."wait"] items=["initialize", "wait", "change sample start", "change sample", "check position", "rotate wheel", "sample change complete", "sample rod up", "sample rod down", "retract rod in", "retract rod out", "insert rod in", "insert rod out", "wheel GV open", "wheel GV close", "vent source", "pump source"]
              }
              frame "rotate wheel" {
                w203 = T8[] [enum."retract rod out", enum."insert rod out", enum."check position", enum."wait"] items=["initialize", "wait", "change sample start", "change sample", "check position", "rotate wheel", "sample change complete", "sample rod up", "sample rod down", "retract rod in", "retract rod out", "insert rod in", "insert rod out", "wheel GV open", "wheel GV close", "vent source", "pump source"]
              }
              frame "change sample" {
                w204 = T8[] [enum."change sample start", enum."sample rod up", enum."retract rod in", enum."retract rod out", enum."check position", enum."insert rod in", enum."insert rod out", enum."sample rod down", enum."sample change complete", enum."wait"] items=["initialize", "wait", "change sample start", "change sample", "check position", "rotate wheel", "sample change complete", "sample rod up", "sample rod down", "retract rod in", "retract rod out", "insert rod in", "insert rod out", "wheel GV open", "wheel GV close", "vent source", "pump source"]
              }
              frame "vent source" {
                w205 = T8[] [enum."sample rod up", enum."retract rod in", enum."retract rod out", enum."insert rod out", enum."wheel GV close", enum."wait"] items=["initialize", "wait", "change sample start", "change sample", "check position", "rotate wheel", "sample change complete", "sample rod up", "sample rod down", "retract rod in", "retract rod out", "insert rod in", "insert rod out", "wheel GV open", "wheel GV close", "vent source", "pump source"]
              }
              frame "pump source" {
                w206 = T8[] [enum."wheel GV open", enum."sample rod up", enum."check position", enum."insert rod in", enum."insert rod out", enum."sample rod down", enum."wait"] items=["initialize", "wait", "change sample start", "change sample", "check position", "rotate wheel", "sample change complete", "sample rod up", "sample rod down", "retract rod in", "retract rod out", "insert rod in", "insert rod out", "wheel GV open", "wheel GV close", "vent source", "pump source"]
              }
              frame "wait", Default {
                w207 = T8[] [enum."wait"] items=["initialize", "wait", "change sample start", "change sample", "check position", "rotate wheel", "sample change complete", "sample rod up", "sample rod down", "retract rod in", "retract rod out", "insert rod in", "insert rod out", "wheel GV open", "wheel GV close", "vent source", "pump source"]
              }
            }
            n114 = shared-variable ".\\local SCA shared var lib.lvlib\\New Command?"(FALSE ("New Command?")) -> ()  [unwired: 1 in, 1 out]
          }
        }
        n115 = Select(t="Ready", s="clear error", f=w189) -> (s? t:f=w188:string)
        n116 = Index Array(array=w185, index=0) -> (element=w184:T8)
        n117 = Tick Count (ms)() -> (millisecond timer value=w183:u32)
      }
      frame "wheel GV open" {
        n118 = shared-variable "SCA-cRIO\\Mod8\\Wheel GV Actuator"(TRUE ("sc gate valve")) -> (error out=w218:errorcluster)  [unwired: 1 in]
        n119 = shared-variable ".\\local SCA shared var lib.lvlib\\Wheel GV Bypass"() -> (w221:bool)  [unwired: 1 in, 1 out]
        n120 = shared-variable "SCA-cRIO\\global SCA shared var lib.lvlib\\Wheel GV Status"(error in=w218) -> (w217:enum16{"status unclear", "closed", "open"})  [unwired: 1 out]
        n121 = Select(t=enum16{"status unclear", "closed", "open"}."open" ("x"), s=w221, f=w217) -> (s? t:f=w216:enum16{"status unclear", "closed", "open"})
        n122 = case shown="\"open\"" w216 {
          tunnel: w215 -> [w228 _]
          tunnel: w210 -> [w227 w235]
          tunnel: w208 -> [w226 w234]
          tunnel: [w225 w233] -> w212
          tunnel: [w224 w232] -> w213
          tunnel: [w223 w231] -> w211
          tunnel: [w222 "wheel GV opened" ("Status Message")] -> w214
          frame "status unclear", "closed", Default {
            n123 = shared-variable ".\\local SCA shared var lib.lvlib\\Wheel GV Timeout"() -> (w229:u32)  [unwired: 1 in, 1 out]
            n124 = call "SCA state Transition Timeout Check.vi"("Start Time"=w228, "Timeout limit"=w229, "Current State In"=w226, "Modified Array of states in"=w227) -> ("Status Message"=w222:string, "millisecond timer value out"=w223:u32, "Next State"=w224:T8, "Modified Array of states out"=w225:T8[])  [unwired: 4 in]
          }
          frame "open" {
            n125 = call "Modify array of SCA states.vi"("Current State"=w234, "Array of states to process"=w235) -> ("Next State"=w232:T8, "Modified Array of states"=w233:T8[])  [unwired: 7 in]
            n126 = Tick Count (ms)() -> (millisecond timer value=w231:u32)
          }
        }
      }
      frame "wheel GV close" {
        n127 = shared-variable "SCA-cRIO\\global SCA shared var lib.lvlib\\Retract Rod Status"() -> (w254:T5)  [unwired: 1 in, 1 out]
        n128 = shared-variable "SCA-cRIO\\global SCA shared var lib.lvlib\\Insert Rod Status"() -> (w252:T5)  [unwired: 1 in, 1 out]
        n129 = shared-variable ".\\local SCA shared var lib.lvlib\\Retract Rod Bypass"() -> (w248:bool)  [unwired: 1 in, 1 out]
        n130 = shared-variable ".\\local SCA shared var lib.lvlib\\Insert Rod Bypass"() -> (w250:bool)  [unwired: 1 in, 1 out]
        n131 = Equal?(x=w252, y=Horizontal_Rod_states."rod out" ("Enum")) -> (x = y?=w251:bool)
        n132 = Equal?(x=w254, y=Horizontal_Rod_states."rod out" ("Enum")) -> (x = y?=w249:bool)
        n133 = Or(x=w250, y=w251) -> (x .or. y?=w247:bool)
        n134 = Or(x=w248, y=w249) -> (x .or. y?=w246:bool)
        n135 = Build Array(w247, w246) -> (w244:bool[])
        n136 = And Array Elements(Boolean array=w244) -> (logical AND=w245:bool)
        n137 = case shown="True" w245 {
          tunnel: w244 -> [w263 _]
          tunnel: w243 -> [w259 w278]
          tunnel: w241 -> [_ w277]
          tunnel: w242 -> [_ w276]
          tunnel: ["wheel GV interlocks not satisfied" ("Status Message") w275] -> w240
          tunnel: [w256 w274] -> w238
          tunnel: [w257 w273] -> w237
          tunnel: [w258 w272] -> w236
          frame False {
            n138 = Search 1D Array(1D array=w263, element=FALSE) -> (index of element=w261:i32)  [unwired: 1 in]
            n139 = case shown="0, Default" w261 {
              tunnel: w259 -> [w264 w271]
              tunnel: [w266 w269] -> w258
              tunnel: [w265 w268] -> w257
              frame 0, Default {
                w265 = SCA_states."insert rod out" ("SC2 state")
                n140 = Insert Into Array(array=w264, index=0, new element=w265) -> (w266:T8[])
              }
              frame 1 {
                w268 = SCA_states."retract rod out" ("SC2 state")
                n141 = Insert Into Array(array=w271, index=0, new element=w268) -> (w269:T8[])
              }
            }
            n142 = Tick Count (ms)() -> (millisecond timer value=w256:u32)
          }
          frame True {
            n143 = shared-variable "SCA-cRIO\\Mod8\\Wheel GV Actuator"(FALSE ("sc gate valve")) -> (error out=w281:errorcluster)  [unwired: 1 in]
            n144 = shared-variable ".\\local SCA shared var lib.lvlib\\Wheel GV Bypass"() -> (w284:bool)  [unwired: 1 in, 1 out]
            n145 = shared-variable "SCA-cRIO\\global SCA shared var lib.lvlib\\Wheel GV Status"(error in=w281) -> (w280:enum16{"status unclear", "closed", "open"})  [unwired: 1 out]
            n146 = Select(t=enum16{"status unclear", "closed", "open"}."closed" ("x"), s=w284, f=w280) -> (s? t:f=w279:enum16{"status unclear", "closed", "open"})
            n147 = case shown="\"status unclear\", \"open\", Default" w279 {
              tunnel: w276 -> [w291 _]
              tunnel: w278 -> [w290 w298]
              tunnel: w277 -> [w289 w297]
              tunnel: [w288 w296] -> w272
              tunnel: [w287 w295] -> w273
              tunnel: [w286 w294] -> w274
              tunnel: [w285 "wheel GV closed" ("Status Message")] -> w275
              frame "status unclear", "open", Default {
                n148 = shared-variable ".\\local SCA shared var lib.lvlib\\Wheel GV Timeout"() -> (w292:u32)  [unwired: 1 in, 1 out]
                n149 = call "SCA state Transition Timeout Check.vi"("Start Time"=w291, "Timeout limit"=w292, "Current State In"=w289, "Modified Array of states in"=w290) -> ("Status Message"=w285:string, "millisecond timer value out"=w286:u32, "Next State"=w287:T8, "Modified Array of states out"=w288:T8[])  [unwired: 4 in]
              }
              frame "closed" {
                n150 = call "Modify array of SCA states.vi"("Current State"=w297, "Array of states to process"=w298) -> ("Next State"=w295:T8, "Modified Array of states"=w296:T8[])  [unwired: 7 in]
                n151 = Tick Count (ms)() -> (millisecond timer value=w294:u32)
              }
            }
          }
        }
      }
      frame "sample rod up" {
        n152 = shared-variable "SCA-cRIO\\Mod8\\Sample Rod Actuator"(FALSE ("Sample Rod Actuator")) -> (error out=w311:errorcluster)  [unwired: 1 in]
        n153 = shared-variable ".\\local SCA shared var lib.lvlib\\Sample Rod Bypass"() -> (w308:bool)  [unwired: 1 in, 1 out]
        n154 = shared-variable "SCA-cRIO\\global SCA shared var lib.lvlib\\Sample Rod status"(error in=w311) -> (w309:T6)  [unwired: 1 out]
        n155 = Select(t=Vertical_Rod_states."rod up" ("y"), s=w308, f=w309) -> (s? t:f=w307:T6)
        n156 = case shown="\"rod up\"" w307 {
          tunnel: w306 -> [w320 w326]
          tunnel: w305 -> [w319 w325]
          tunnel: w304 -> [w318 _]
          tunnel: [w314 "sample rod up" ("Status Message")] -> w302
          tunnel: [w315 w323] -> w301
          tunnel: [w316 w322] -> w300
          tunnel: [w317 w321] -> w299
          frame "status unclear", "rod down", Default {
            n157 = shared-variable ".\\local SCA shared var lib.lvlib\\Sample Rod Timeout"() -> (w313:u32)  [unwired: 1 in, 1 out]
            n158 = call "SCA state Transition Timeout Check.vi"("Start Time"=w318, "Timeout limit"=w313, "Current State In"=w319, "Modified Array of states in"=w320) -> ("Status Message"=w314:string, "millisecond timer value out"=w315:u32, "Next State"=w316:T8, "Modified Array of states out"=w317:T8[])  [unwired: 4 in]
          }
          frame "rod up" {
            n159 = call "Modify array of SCA states.vi"("Current State"=w325, "Array of states to process"=w326) -> ("Next State"=w322:T8, "Modified Array of states"=w321:T8[])  [unwired: 7 in]
            n160 = Tick Count (ms)() -> (millisecond timer value=w323:u32)
          }
        }
      }
      frame "sample rod down" {
        n161 = shared-variable "SCA-cRIO\\global SCA shared var lib.lvlib\\Retract Rod Status"() -> (w345:T5)  [unwired: 1 in, 1 out]
        n162 = shared-variable "SCA-cRIO\\global SCA shared var lib.lvlib\\Insert Rod Status"() -> (w343:T5)  [unwired: 1 in, 1 out]
        n163 = shared-variable ".\\local SCA shared var lib.lvlib\\Retract Rod Bypass"() -> (w339:bool)  [unwired: 1 in, 1 out]
        n164 = shared-variable ".\\local SCA shared var lib.lvlib\\Insert Rod Bypass"() -> (w341:bool)  [unwired: 1 in, 1 out]
        n165 = Equal?(x=w343, y=Horizontal_Rod_states."rod out" ("Enum")) -> (x = y?=w342:bool)
        n166 = Equal?(x=w345, y=Horizontal_Rod_states."rod out" ("Enum")) -> (x = y?=w340:bool)
        n167 = Or(x=w341, y=w342) -> (x .or. y?=w338:bool)
        n168 = Or(x=w339, y=w340) -> (x .or. y?=w337:bool)
        n169 = Build Array(w338, w337) -> (w335:bool[])
        n170 = And Array Elements(Boolean array=w335) -> (logical AND=w336:bool)
        n171 = case shown="True" w336 {
          tunnel: w335 -> [w354 _]
          tunnel: w334 -> [w350 w370]
          tunnel: w333 -> [_ w369]
          tunnel: w332 -> [_ w368]
          tunnel: ["sample rod down interlocks not satisfied" ("Status Message") w367] -> w331
          tunnel: [w347 w366] -> w329
          tunnel: [w348 w365] -> w328
          tunnel: [w349 w364] -> w327
          frame False {
            n172 = Search 1D Array(1D array=w354, element=FALSE) -> (index of element=w352:i32)  [unwired: 1 in]
            n173 = case shown="0, Default" w352 {
              tunnel: w350 -> [w355 w362]
              tunnel: [w357 w360] -> w349
              tunnel: [w356 w359] -> w348
              frame 0, Default {
                w356 = SCA_states."insert rod out" ("SC2 state")
                n174 = Insert Into Array(array=w355, index=0, new element=w356) -> (w357:T8[])
              }
              frame 1 {
                w359 = SCA_states."retract rod out" ("SC2 state")
                n175 = Insert Into Array(array=w362, index=0, new element=w359) -> (w360:T8[])
              }
            }
            n176 = Tick Count (ms)() -> (millisecond timer value=w347:u32)
          }
          frame True {
            n177 = shared-variable "SCA-cRIO\\Mod8\\Sample Rod Actuator"(TRUE ("sc gate valve")) -> (error out=w373:errorcluster)  [unwired: 1 in]
            n178 = shared-variable ".\\local SCA shared var lib.lvlib\\Sample Rod Bypass"() -> (w375:bool)  [unwired: 1 in, 1 out]
            n179 = shared-variable "SCA-cRIO\\global SCA shared var lib.lvlib\\Sample Rod status"(error in=w373) -> (w372:T6)  [unwired: 1 out]
            n180 = Select(t=Vertical_Rod_states."rod up" ("y"), s=w375, f=w372) -> (s? t:f=w371:T6)
            n181 = case shown="\"status unclear\", \"rod up\", Default" w371 {
              tunnel: w368 -> [w382 _]
              tunnel: w370 -> [w381 w389]
              tunnel: w369 -> [w380 w388]
              tunnel: [w379 w387] -> w364
              tunnel: [w378 w386] -> w365
              tunnel: [w377 w385] -> w366
              tunnel: [w376 "sample rod down" ("Status Message")] -> w367
              frame "status unclear", "rod up", Default {
                n182 = shared-variable ".\\local SCA shared var lib.lvlib\\Sample Rod Timeout"() -> (w383:u32)  [unwired: 1 in, 1 out]
                n183 = call "SCA state Transition Timeout Check.vi"("Start Time"=w382, "Timeout limit"=w383, "Current State In"=w380, "Modified Array of states in"=w381) -> ("Status Message"=w376:string, "millisecond timer value out"=w377:u32, "Next State"=w378:T8, "Modified Array of states out"=w379:T8[])  [unwired: 4 in]
              }
              frame "rod down" {
                n184 = call "Modify array of SCA states.vi"("Current State"=w388, "Array of states to process"=w389) -> ("Next State"=w386:T8, "Modified Array of states"=w387:T8[])  [unwired: 7 in]
                n185 = Tick Count (ms)() -> (millisecond timer value=w385:u32)
              }
            }
          }
        }
      }
      frame "retract rod in" {
        n186 = shared-variable "SCA-cRIO\\global SCA shared var lib.lvlib\\Sample Rod status"() -> (w394:T6)  [unwired: 1 in, 1 out]
        n187 = shared-variable "SCA-cRIO\\global SCA shared var lib.lvlib\\Insert Rod Status"() -> (w412:T5)  [unwired: 1 in, 1 out]
        n188 = shared-variable "SCA-cRIO\\global SCA shared var lib.lvlib\\Wheel GV Status"() -> (w414:enum16{"status unclear", "closed", "open"})  [unwired: 1 in, 1 out]
        n189 = shared-variable ".\\local SCA shared var lib.lvlib\\Wheel GV Bypass"() -> (w408:bool)  [unwired: 1 in, 1 out]
        n190 = shared-variable ".\\local SCA shared var lib.lvlib\\Sample Rod Bypass"() -> (w392:bool)  [unwired: 1 in, 1 out]
        n191 = shared-variable ".\\local SCA shared var lib.lvlib\\Insert Rod Bypass"() -> (w410:bool)  [unwired: 1 in, 1 out]
        n192 = Equal?(x=w412, y=Horizontal_Rod_states."rod out" ("Enum")) -> (x = y?=w411:bool)
        n193 = Equal?(x=w414, y=enum16{"status unclear", "closed", "open"}."open") -> (x = y?=w409:bool)
        n194 = Equal?(x=w394, y=Vertical_Rod_states."rod up") -> (x = y?=w393:bool)
        n195 = Or(x=w410, y=w411) -> (x .or. y?=w407:bool)
        n196 = Or(x=w408, y=w409) -> (x .or. y?=w406:bool)
        n197 = Or(x=w392, y=w393) -> (x .or. y?=w391:bool)
        n198 = Build Array(w407, w406, w391) -> (w404:bool[])
        n199 = And Array Elements(Boolean array=w404) -> (logical AND=w405:bool)
        n200 = case shown="True" w405 {
          tunnel: w404 -> [w422 _]
          tunnel: w403 -> [w418 w442]
          tunnel: w402 -> [_ w441]
          tunnel: w401 -> [_ w440]
          tunnel: ["retract rod in interlocks not satisfied" ("Status Message") w439] -> w399
          tunnel: [w415 w438] -> w398
          tunnel: [w416 w437] -> w397
          tunnel: [w417 w436] -> w396
          frame False {
            n201 = Search 1D Array(1D array=w422, element=FALSE) -> (index of element=w420:i32)  [unwired: 1 in]
            n202 = case shown="0, Default" w420 {
              tunnel: w418 -> [w423 w430 w434]
              tunnel: [w425 w428 w432] -> w417
              tunnel: [w424 w427 w431] -> w416
              frame 0, Default {
                w424 = SCA_states."insert rod out" ("SC2 state")
                n203 = Insert Into Array(array=w423, index=0, new element=w424) -> (w425:T8[])
              }
              frame 1 {
                w427 = SCA_states."wheel GV open" ("SC2 state")
                n204 = Insert Into Array(array=w430, index=0, new element=w427) -> (w428:T8[])
              }
              frame 2 {
                w431 = SCA_states."sample rod up" ("SC2 state")
                n205 = Insert Into Array(array=w434, index=0, new element=w431) -> (w432:T8[])
              }
            }
            n206 = Tick Count (ms)() -> (millisecond timer value=w415:u32)
          }
          frame True {
            n207 = shared-variable "SCA-cRIO\\Mod8\\Retract Rod Actuator"(TRUE ("sc gate valve")) -> (error out=w445:errorcluster)  [unwired: 1 in]
            n208 = shared-variable ".\\local SCA shared var lib.lvlib\\Retract Rod Bypass"() -> (w447:bool)  [unwired: 1 in, 1 out]
            n209 = shared-variable "SCA-cRIO\\global SCA shared var lib.lvlib\\Retract Rod Status"(error in=w445) -> (w444:T5)  [unwired: 1 out]
            n210 = Select(t=Horizontal_Rod_states."rod in", s=w447, f=w444) -> (s? t:f=w443:T5)
            n211 = case shown="\"rod in\"" w443 {
              tunnel: w440 -> [w454 _]
              tunnel: w442 -> [w453 w461]
              tunnel: w441 -> [w452 w460]
              tunnel: [w451 w459] -> w436
              tunnel: [w450 w458] -> w437
              tunnel: [w449 w457] -> w438
              tunnel: [w448 "retract rod in" ("Status Message")] -> w439
              frame "status unclear", "rod out", Default {
                n212 = shared-variable ".\\local SCA shared var lib.lvlib\\Retract Rod Timeout"() -> (w455:u32)  [unwired: 1 in, 1 out]
                n213 = call "SCA state Transition Timeout Check.vi"("Start Time"=w454, "Timeout limit"=w455, "Current State In"=w452, "Modified Array of states in"=w453) -> ("Status Message"=w448:string, "millisecond timer value out"=w449:u32, "Next State"=w450:T8, "Modified Array of states out"=w451:T8[])  [unwired: 4 in]
              }
              frame "rod in" {
                n214 = call "Modify array of SCA states.vi"("Current State"=w460, "Array of states to process"=w461) -> ("Next State"=w458:T8, "Modified Array of states"=w459:T8[])  [unwired: 7 in]
                n215 = Tick Count (ms)() -> (millisecond timer value=w457:u32)
              }
            }
          }
        }
      }
      frame "retract rod out" {
        n216 = shared-variable "SCA-cRIO\\Mod8\\Retract Rod Actuator"(FALSE ("Sample Rod Actuator")) -> (error out=w474:errorcluster)  [unwired: 1 in]
        n217 = shared-variable ".\\local SCA shared var lib.lvlib\\Retract Rod Bypass"() -> (w473:bool)  [unwired: 1 in, 1 out]
        n218 = shared-variable "SCA-cRIO\\global SCA shared var lib.lvlib\\Retract Rod Status"(error in=w474) -> (w471:T5)  [unwired: 1 out]
        n219 = Select(t=Horizontal_Rod_states."rod out" ("Enum"), s=w473, f=w471) -> (s? t:f=w470:T5)
        n220 = case shown="\"rod out\"" w470 {
          tunnel: w469 -> [w482 w489]
          tunnel: w468 -> [w481 w488]
          tunnel: w467 -> [w480 _]
          tunnel: [w476 "retract rod out" ("Status Message")] -> w465
          tunnel: [w479 w486] -> w464
          tunnel: [w478 w485] -> w463
          tunnel: [w477 w484] -> w462
          frame "status unclear", "rod in", Default {
            n221 = shared-variable ".\\local SCA shared var lib.lvlib\\Retract Rod Timeout"() -> (w483:u32)  [unwired: 1 in, 1 out]
            n222 = call "SCA state Transition Timeout Check.vi"("Start Time"=w480, "Timeout limit"=w483, "Current State In"=w481, "Modified Array of states in"=w482) -> ("Status Message"=w476:string, "millisecond timer value out"=w479:u32, "Next State"=w478:T8, "Modified Array of states out"=w477:T8[])  [unwired: 4 in]
          }
          frame "rod out" {
            n223 = call "Modify array of SCA states.vi"("Current State"=w488, "Array of states to process"=w489) -> ("Next State"=w485:T8, "Modified Array of states"=w484:T8[])  [unwired: 7 in]
            n224 = Tick Count (ms)() -> (millisecond timer value=w486:u32)
          }
        }
      }
      frame "insert rod in" {
        n225 = shared-variable "SCA-cRIO\\global SCA shared var lib.lvlib\\Retract Rod Status"() -> (w512:T5)  [unwired: 1 in, 1 out]
        n226 = shared-variable "SCA-cRIO\\global SCA shared var lib.lvlib\\Sample Rod status"() -> (w502:T6)  [unwired: 1 in, 1 out]
        n227 = shared-variable "SCA-cRIO\\global SCA shared var lib.lvlib\\Wheel GV Status"() -> (w514:enum16{"status unclear", "closed", "open"})  [unwired: 1 in, 1 out]
        n228 = shared-variable ".\\local SCA shared var lib.lvlib\\Wheel GV Bypass"() -> (w508:bool)  [unwired: 1 in, 1 out]
        n229 = shared-variable ".\\local SCA shared var lib.lvlib\\Sample Rod Bypass"() -> (w500:bool)  [unwired: 1 in, 1 out]
        n230 = shared-variable ".\\local SCA shared var lib.lvlib\\Retract Rod Bypass"() -> (w510:bool)  [unwired: 1 in, 1 out]
        n231 = Equal?(x=w512, y=Horizontal_Rod_states."rod out" ("Enum")) -> (x = y?=w511:bool)
        n232 = Equal?(x=w514, y=enum16{"status unclear", "closed", "open"}."open") -> (x = y?=w509:bool)
        n233 = Equal?(x=w502, y=Vertical_Rod_states."rod up") -> (x = y?=w501:bool)
        n234 = Or(x=w510, y=w511) -> (x .or. y?=w507:bool)
        n235 = Or(x=w508, y=w509) -> (x .or. y?=w506:bool)
        n236 = Or(x=w500, y=w501) -> (x .or. y?=w499:bool)
        n237 = Build Array(w507, w506, w499) -> (w504:bool[])
        n238 = And Array Elements(Boolean array=w504) -> (logical AND=w505:bool)
        n239 = case shown="False" w505 {
          tunnel: w504 -> [w522 _]
          tunnel: w497 -> [w518 w542]
          tunnel: w496 -> [_ w541]
          tunnel: w495 -> [_ w540]
          tunnel: ["retract rod in interlocks not satisfied" ("Status Message") w539] -> w494
          tunnel: [w515 w538] -> w490
          tunnel: [w516 w537] -> w491
          tunnel: [w517 w536] -> w492
          frame False {
            n240 = Search 1D Array(1D array=w522, element=FALSE) -> (index of element=w520:i32)  [unwired: 1 in]
            n241 = case shown="2" w520 {
              tunnel: w518 -> [w523 w530 w534]
              tunnel: [w525 w528 w532] -> w517
              tunnel: [w524 w527 w531] -> w516
              frame 0, Default {
                w524 = SCA_states."retract rod out" ("SC2 state")
                n242 = Insert Into Array(array=w523, index=0, new element=w524) -> (w525:T8[])
              }
              frame 1 {
                w527 = SCA_states."wheel GV open" ("SC2 state")
                n243 = Insert Into Array(array=w530, index=0, new element=w527) -> (w528:T8[])
              }
              frame 2 {
                w531 = SCA_states."sample rod up" ("SC2 state")
                n244 = Insert Into Array(array=w534, index=0, new element=w531) -> (w532:T8[])
              }
            }
            n245 = Tick Count (ms)() -> (millisecond timer value=w515:u32)
          }
          frame True {
            n246 = shared-variable "SCA-cRIO\\Mod8\\Insert Rod Actuator"(TRUE ("sc gate valve")) -> (error out=w545:errorcluster)  [unwired: 1 in]
            n247 = shared-variable ".\\local SCA shared var lib.lvlib\\Insert Rod Bypass"() -> (w547:bool)  [unwired: 1 in, 1 out]
            n248 = shared-variable "SCA-cRIO\\global SCA shared var lib.lvlib\\Insert Rod Status"(error in=w545) -> (w544:T5)  [unwired: 1 out]
            n249 = Select(t=Horizontal_Rod_states."rod in", s=w547, f=w544) -> (s? t:f=w543:T5)
            n250 = case shown="\"status unclear\", \"rod out\", Default" w543 {
              tunnel: w540 -> [w554 _]
              tunnel: w542 -> [w553 w561]
              tunnel: w541 -> [w552 w560]
              tunnel: [w551 w559] -> w536
              tunnel: [w550 w558] -> w537
              tunnel: [w549 w557] -> w538
              tunnel: [w548 "insert rod in" ("Status Message")] -> w539
              frame "status unclear", "rod out", Default {
                n251 = shared-variable ".\\local SCA shared var lib.lvlib\\Insert Rod Timeout"() -> (w555:u32)  [unwired: 1 in, 1 out]
                n252 = call "SCA state Transition Timeout Check.vi"("Start Time"=w554, "Timeout limit"=w555, "Current State In"=w552, "Modified Array of states in"=w553) -> ("Status Message"=w548:string, "millisecond timer value out"=w549:u32, "Next State"=w550:T8, "Modified Array of states out"=w551:T8[])  [unwired: 4 in]
              }
              frame "rod in" {
                n253 = call "Modify array of SCA states.vi"("Current State"=w560, "Array of states to process"=w561) -> ("Next State"=w558:T8, "Modified Array of states"=w559:T8[])  [unwired: 7 in]
                n254 = Tick Count (ms)() -> (millisecond timer value=w557:u32)
              }
            }
          }
        }
      }
      frame "insert rod out" {
        n255 = shared-variable "SCA-cRIO\\Mod8\\Insert Rod Actuator"(FALSE ("Sample Rod Actuator")) -> (error out=w574:errorcluster)  [unwired: 1 in]
        n256 = shared-variable ".\\local SCA shared var lib.lvlib\\Insert Rod Bypass"() -> (w573:bool)  [unwired: 1 in, 1 out]
        n257 = shared-variable "SCA-cRIO\\global SCA shared var lib.lvlib\\Insert Rod Status"(error in=w574) -> (w562:T5)  [unwired: 1 out]
        n258 = Select(t=Horizontal_Rod_states."rod out" ("Enum"), s=w573, f=w562) -> (s? t:f=w571:T5)
        n259 = case shown="\"rod out\"" w571 {
          tunnel: w570 -> [w582 w589]
          tunnel: w569 -> [w581 w588]
          tunnel: w568 -> [w580 _]
          tunnel: [w576 "insert rod out" ("Status Message")] -> w563
          tunnel: [w579 w586] -> w566
          tunnel: [w578 w585] -> w565
          tunnel: [w577 w584] -> w564
          frame "status unclear", "rod in", Default {
            n260 = shared-variable ".\\local SCA shared var lib.lvlib\\Insert Rod Timeout"() -> (w583:u32)  [unwired: 1 in, 1 out]
            n261 = call "SCA state Transition Timeout Check.vi"("Start Time"=w580, "Timeout limit"=w583, "Current State In"=w581, "Modified Array of states in"=w582) -> ("Status Message"=w576:string, "millisecond timer value out"=w579:u32, "Next State"=w578:T8, "Modified Array of states out"=w577:T8[])  [unwired: 4 in]
          }
          frame "rod out" {
            n262 = call "Modify array of SCA states.vi"("Current State"=w588, "Array of states to process"=w589) -> ("Next State"=w585:T8, "Modified Array of states"=w584:T8[])  [unwired: 7 in]
            n263 = Tick Count (ms)() -> (millisecond timer value=w586:u32)
          }
        }
      }
      frame "change sample start" {
        n264 = call "Modify array of SCA states.vi"("Current State"=w592, "Array of states to process"=w594) -> ("Next State"=w590:T8, "Modified Array of states"=w593:T8[])  [unwired: 7 in]
        n265 = shared-variable ".\\local SCA shared var lib.lvlib\\Changing Sample"(TRUE ("Changing Sample")) -> ()  [unwired: 1 in, 1 out]
        n266 = Select(t="Ready", s="clear error 2", f=w598) -> (s? t:f=w591:string)
        n267 = Tick Count (ms)() -> (millisecond timer value=w595:u32)
      }
      frame "rotate wheel" {
        w614 = 10000.0 ("acceleration")
        # "in motor steps"
        # "The counter logic here (along with \"wait position\") doesn't appear to have a clear purpose.  Doesn't appear that the failure state could ever be acheived as the max timer"
        n268 = shared-variable ".\\local SCA shared var lib.lvlib\\Motor Status"(FALSE ("Motor Status")) -> (error out=w601:errorcluster)  [unwired: 1 in]
        n269 = shared-variable "SCA-cRIO\\global SCA shared var lib.lvlib\\New Move"() -> (w610:dbl)  [unwired: 1 in, 1 out]
        n270 = shared-variable ".\\local SCA shared var lib.lvlib\\Execute Move"(error in=w601) -> (w605:bool)  [unwired: 1 out]
        n271 = xnode "Straight-Line Move"("resource"=w615, "execute"=w605, "position"=w610, "velocity"=w614, "acceleration"=w614, "deceleration"=w614, "accel. jerk"=w614, "smoothing"=w614) -> ("error out"=→"Rotate Wheel error":errorcluster, "done"=w613:bool)  [unwired: 2 in, 4 out]
        "Rotation done" <- w613
        n272 = Not(x=w613) -> (.not. x?=w602:bool)
        n273 = shared-variable ".\\local SCA shared var lib.lvlib\\Execute Move"(w602) -> ()  [unwired: 1 in, 1 out]
        n274 = Select(t=SCA_states."check position" ("SC2 state"), s=w613, f=SCA_states."rotate wheel" ("SC2 state")) -> (s? t:f=w603:T8)
      }
      frame "check position" {
        n275 = Tick Count (ms)() -> (millisecond timer value=w645:u32)
        n276 = shared-variable ".\\local SCA shared var lib.lvlib\\Rotate Wheel timeout"() -> (w650:u32)  [unwired: 1 in, 1 out]
        n277 = shared-variable ".\\local SCA shared var lib.lvlib\\Rotate Wheel Minimum Time"() -> (w647:u32)  [unwired: 1 in, 1 out]
        n278 = Subtract(x=w645, y=w648) -> (x-y=w649:u32)
        n279 = Greater?(x=w650, y=w649) -> (0:w642:bool)
        n280 = Subtract(x=w645, y=w651) -> (x-y=w646:u32)
        n281 = Less?(x=w647, y=w646) -> (x < y?=w644:bool)
        n282 = And(x=w642, y=w644) -> (x .and. y?=w643:bool)
        n283 = case shown="True" w643 {
          tunnel: w659 -> [w664 w683]
          tunnel: [w661 w682] -> w658
          tunnel: [w660 w681] -> w657
          tunnel: [w663 w680] -> w656
          tunnel: w655 -> [_ w679]
          tunnel: w654 -> [w665 w678]
          tunnel: [w662 w677] -> w653
          tunnel: [w666 w676] -> w652
          tunnel: w651 -> [w660 w675]
          tunnel: w648 -> [w661 w674]
          tunnel: w642 -> [w667 _]
          frame False {
            n284 = case shown="False" w667 {
              tunnel: ["Wheel rotation timed out" "waiting to check position"] -> w666
              tunnel: w665 -> [_ w671]
              tunnel: w664 -> [_ w672]
              tunnel: [SCA_states."wait" ("SC2 state") w672] -> w663
              tunnel: [w668 w671] -> w662
              frame False {
                w668 = T8[] [enum."wait"] items=["initialize", "wait", "change sample start", "change sample", "check position", "rotate wheel", "sample change complete", "sample rod up", "sample rod down", "retract rod in", "retract rod out", "insert rod in", "insert rod out", "wheel GV open", "wheel GV close", "vent source", "pump source"]
                # "Timeout reached"
              }
              frame True {
                # "Haven't met minimum wait time yet"
              }
            }
          }
          frame True {
            # "Move in motor steps"
            n285 = shared-variable "SCA-cRIO\\global SCA shared var lib.lvlib\\Encoder position"() -> (w695:i16)  [unwired: 1 in, 1 out]
            n286 = shared-variable "SCA-cRIO\\global SCA shared var lib.lvlib\\Encoder Offset"() -> (w696:i16)  [unwired: 1 in, 1 out]
            n287 = shared-variable ".\\local SCA shared var lib.lvlib\\New sample"() -> (w692:i8)  [unwired: 1 in, 1 out]
            n288 = call "SCA Sample-Encoder conversion.vi"("Step Window Radius"="Step Window Radius", "Rollover Sample"="Rollover Sample", "Encoder Offset"=w695, "Encoder Position"=w696, "Desired Sample"=w692) -> ("Window limit 1"=→"Window Limit 1":i16, "Within Range?"=w684:bool, "Encoder destination"=w697:i16, "Window limit 2"=→"Window Limit 2":i16, "New move (encoder steps)"=w689:i16)  [unwired: 2 in]
            "Encoder Destination" <- w697
            "In Range?" <- w684
            n289 = To Double Precision Float(number=w689) -> (double precision float=w685:dbl)
            n290 = Divide(x=50000.0, y=16384.0) -> (x/y=w688:dbl)
            n291 = shared-variable "SCA-cRIO\\global SCA shared var lib.lvlib\\Encoder Destination"(w697) -> ()  [unwired: 1 in, 1 out]
            n292 = shared-variable ".\\local SCA shared var lib.lvlib\\Motor Status"(w684) -> ()  [unwired: 1 in, 1 out]
            n293 = Multiply(x=w688, y=w685) -> (x*y=w698:dbl)
            "New Move" <- w698
            n294 = shared-variable "SCA-cRIO\\global SCA shared var lib.lvlib\\New Move"(w698) -> ()  [unwired: 1 in, 1 out]
            n295 = case shown="False" w684 {
              tunnel: [SCA_states."rotate wheel" ("SC2 state") w711] -> w680
              tunnel: ["rotating sample wheel" "rotation complete"] -> w676
              tunnel: [w699 w710] -> w677
              tunnel: [w700 w704] -> w681
              tunnel: [w701 w704] -> w682
              tunnel: w675 -> [_ _]
              tunnel: w674 -> [w701 _]
              tunnel: w683 -> [_ w709]
              tunnel: w678 -> [w699 w708]
              tunnel: w679 -> [_ w706]
              frame False {
                # "wheel not in correct position, rotate again"
                n296 = Tick Count (ms)() -> (millisecond timer value=w700:u32)
              }
              frame True {
                n297 = call "Modify array of SCA states.vi"("Current State"=w709, "Array of states to process"=w708) -> ("Next State"=w711:T8, "Modified Array of states"=w710:T8[])  [unwired: 7 in]
                n298 = xnode "Straight-Line Move"("resource"=w706, "execute"=FALSE) -> ()  [unwired: 8 in, 6 out]
                n299 = Tick Count (ms)() -> (millisecond timer value=w704:u32)
              }
            }
          }
        }
      }
      frame "sample change complete" {
        n300 = call "Modify array of SCA states.vi"("Current State"=w740, "Array of states to process"=w741) -> ("Next State"=w738:T8, "Modified Array of states"=w739:T8[])  [unwired: 7 in]
        n301 = shared-variable ".\\local SCA shared var lib.lvlib\\Changing Sample"(FALSE ("Changing Sample")) -> (error out=w742:errorcluster)  [unwired: 1 in]
        n302 = Select(t="Ready", s="clear error 3", f=w748) -> (s? t:f=w747:string)
        n303 = Tick Count (ms)() -> (millisecond timer value=w744:u32)
        n304 = shared-variable ".\\local SCA shared var lib.lvlib\\Motor Status"(TRUE ("Motor Status"), error in=w742) -> ()  [unwired: 1 out]
      }
    }
    "action" <- w157
    "SCA next state" <- w155
    n305 = shared-variable "SCA-cRIO\\global SCA shared var lib.lvlib\\Status Message"(w160) -> ()  [unwired: 1 in, 1 out]
    n306 = call "Wait Until Next Multiple"("Count(mSec)"=u32 5) -> ()  [unwired: 1 out]
  }
  n307 = while {
    shift-right: [w754] -> _
    shift-left: timestamp(0 s since 1904-01-01) -> [w753]
    stop <- FALSE stop-if-true
    # "SCA command monitor -- when timestamp updated, new command processed"
    n308 = shared-variable "SCA-cRIO\\global SCA shared var lib.lvlib\\SCA Command"() -> (w750:T3, w755:timestamp)  [unwired: 1 in, 1 out]
    "SCA Command" <- w750
    n309 = Wait Until Next ms Multiple(millisecond multiple=u32 50) -> ()  [unwired: 1 out]
    n310 = Equal?(x=w755, y=w753) -> (x = y?=w756:bool)
    n311 = case shown="False" w756 {
      tunnel: w755 -> [w761 _]
      tunnel: [w761 w802] -> w754
      tunnel: w753 -> [_ w802]
      tunnel: w750 -> [w760 _]
      frame False {
        n312 = case shown="\"Start random sample change\"" w760 {
          tunnel: [SCA_states."insert rod out" ("SC2 state") SCA_states."insert rod in" ("SC2 state") SCA_states."retract rod out" ("SC2 state") SCA_states."retract rod in" ("SC2 state") SCA_states."sample rod up" ("SC2 state") SCA_states."sample rod down" ("SC2 state") SCA_states."wheel GV open" ("SC2 state") SCA_states."wheel GV close" ("SC2 state") SCA_states."wait" ("SC2 state") SCA_states."wait" ("SC2 state") SCA_states."pump source" ("SC2 state") SCA_states."vent source" ("SC2 state") w775 w780 w789 w793] -> w759
          frame "Retract insert rod", Default {
          }
          frame "Insert insert rod" {
          }
          frame "Retract retract rod" {
          }
          frame "Insert retract rod" {
          }
          frame "Retract sample rod" {
          }
          frame "Insert sample rod" {
          }
          frame "Open wheel GV" {
          }
          frame "Close wheel GV" {
          }
          frame "Open ion source GV" {
          }
          frame "Close ion source GV" {
          }
          frame "Pump out source" {
          }
          frame "Vent source" {
          }
          frame "Rotate wheel" {
            n313 = shared-variable ".\\local SCA shared var lib.lvlib\\Motor Status"() -> (w774:bool)  [unwired: 1 in, 1 out]
            n314 = case shown="True" w774 {
              tunnel: [SCA_states."wait" ("SC2 state") SCA_states."rotate wheel" ("SC2 state")] -> w775
              frame False {
              }
              frame True {
                n315 = shared-variable "SCA-cRIO\\global SCA shared var lib.lvlib\\Requested Sample"() -> (w777:u8)  [unwired: 1 in, 1 out]
                n316 = shared-variable ".\\local SCA shared var lib.lvlib\\New sample"(w777) -> ()  [unwired: 1 in, 1 out]
              }
            }
          }
          frame "Rotate wheel randomly" {
            n317 = shared-variable ".\\local SCA shared var lib.lvlib\\Motor Status"() -> (w779:bool)  [unwired: 1 in, 1 out]
            n318 = case shown="True" w779 {
              tunnel: [SCA_states."wait" ("SC2 state") SCA_states."rotate wheel" ("SC2 state")] -> w780
              frame False {
              }
              frame True {
                n319 = Random Number (0-1)() -> (number: 0 to 1=w785:dbl)
                n320 = Multiply(x=w785, y=63.0) -> (x*y=w783:dbl)
                n321 = Round Toward +Infinity(x=w783) -> (ceil(x): smallest int >= x=w786:dbl)
                n322 = To Unsigned Byte Integer(number=w786) -> (unsigned 8bit integer=w782:u8)
                n323 = shared-variable ".\\local SCA shared var lib.lvlib\\New sample"(w782) -> ()  [unwired: 1 in, 1 out]
              }
            }
          }
          frame "Start sample change" {
            n324 = shared-variable ".\\local SCA shared var lib.lvlib\\Motor Status"() -> (w788:bool)  [unwired: 1 in, 1 out]
            n325 = case shown="False" w788 {
              tunnel: [SCA_states."wait" ("SC2 state") SCA_states."change sample" ("SC2 state")] -> w789
              frame False {
              }
              frame True {
                n326 = shared-variable "SCA-cRIO\\global SCA shared var lib.lvlib\\Requested Sample"() -> (w791:u8)  [unwired: 1 in, 1 out]
                n327 = shared-variable ".\\local SCA shared var lib.lvlib\\New sample"(w791) -> ()  [unwired: 1 in, 1 out]
              }
            }
          }
          frame "Start random sample change" {
            n328 = shared-variable ".\\local SCA shared var lib.lvlib\\Motor Status"() -> (w794:bool)  [unwired: 1 in, 1 out]
            n329 = case shown="True" w794 {
              tunnel: [SCA_states."wait" ("SC2 state") SCA_states."change sample" ("SC2 state")] -> w793
              frame False {
              }
              frame True {
                n330 = Random Number (0-1)() -> (number: 0 to 1=w799:dbl)
                n331 = Multiply(x=w799, y=63.0) -> (x*y=w797:dbl)
                n332 = Round Toward +Infinity(x=w797) -> (ceil(x): smallest int >= x=w800:dbl)
                n333 = To Unsigned Byte Integer(number=w800) -> (unsigned 8bit integer=w796:u8)
                n334 = shared-variable ".\\local SCA shared var lib.lvlib\\New sample"(w796) -> ()  [unwired: 1 in, 1 out]
              }
            }
          }
        }
        n335 = shared-variable ".\\local SCA shared var lib.lvlib\\SCA state control"(w759) -> (error out=w757:errorcluster)  [unwired: 1 in]
        n336 = shared-variable ".\\local SCA shared var lib.lvlib\\New Command?"(TRUE ("New Command?"), error in=w757) -> ()  [unwired: 1 out]
      }
      frame True {
      }
    }
  }
  n337 = node-c288() -> (w6:T12)  [unwired: 4 in]
  n338 = while {
    shift-right: [w819] -> _
    shift-left: 0.0 ("AI1") -> [w822]
    shift-right: [w817] -> _
    shift-left: w3 -> [w816]
    shift-right: [w818] -> _
    shift-left: w3 -> [w815]
    shift-right: [w813] -> _
    shift-left: w3 -> [w812]
    shift-right: [w810] -> _
    shift-left: w3 -> [w809]
    shift-right: [w804] -> _
    shift-left: w3 -> [w807]
    shift-right: [w803] -> _
    shift-left: w3 -> [w808]
    stop <- FALSE stop-if-true
    # "HV readback loop"
    n339 = shared-variable "SCA-cRIO\\Mod5\\Immersion Lens V read"() -> (w805:dbl)  [unwired: 1 in, 1 out]
    n340 = shared-variable "SCA-cRIO\\Mod5\\Immersion Lens I read"() -> (w806:dbl)  [unwired: 1 in, 1 out]
    n341 = Wait Until Next ms Multiple(millisecond multiple=u32 10) -> ()  [unwired: 1 out]
    n342 = Greater Or Equal?(x=w822, y=100.0) -> (x >= y?=w820:bool)
    n343 = shared-variable "SCA-cRIO\\Mod5\\Extractor V read"() -> (w814:dbl)  [unwired: 1 in, 1 out]
    n344 = shared-variable "SCA-cRIO\\Mod5\\Extractor I read"() -> (w811:dbl)  [unwired: 1 in, 1 out]
    n345 = shared-variable "SCA-cRIO\\Mod5\\Cathode V read"() -> (w824:dbl)  [unwired: 1 in, 1 out]
    n346 = shared-variable "SCA-cRIO\\Mod5\\Cathode I read"() -> (w823:dbl)  [unwired: 1 in, 1 out]
    n347 = case shown="True" w820 {
      tunnel: w824 -> [w842 _]
      tunnel: w823 -> [w843 _]
      tunnel: w822 -> [w846 _]
      tunnel: [w845 0.0 ("AI1")] -> w819
      tunnel: [w844 w850] -> w818
      tunnel: [w841 w850] -> w817
      tunnel: w816 -> [w840 w858]
      tunnel: w815 -> [w839 w859]
      tunnel: w814 -> [w838 _]
      tunnel: [w837 w850] -> w813
      tunnel: w812 -> [w836 w857]
      tunnel: w811 -> [w835 _]
      tunnel: [w834 w850] -> w810
      tunnel: w809 -> [w833 w856]
      tunnel: w808 -> [w832 w849]
      tunnel: w807 -> [w831 w848]
      tunnel: w806 -> [w830 _]
      tunnel: w805 -> [w829 _]
      tunnel: [w828 w850] -> w804
      tunnel: [w827 w850] -> w803
      frame False {
        n348 = Build Array (concatenate)(w830, w831) -> (w828:dbl[])
        n349 = Build Array (concatenate)(w829, w832) -> (w827:dbl[])
        n350 = Build Array (concatenate)(w843, w839) -> (w844:dbl[])
        n351 = Build Array (concatenate)(w842, w840) -> (w841:dbl[])
        n352 = Build Array (concatenate)(w838, w836) -> (w837:dbl[])
        n353 = Build Array (concatenate)(w835, w833) -> (w834:dbl[])
        n354 = Increment(x=w846) -> (x+1=w845:dbl)
      }
      frame True {
        w850 = dbl[] []
        n355 = call-poly <vilib>:"Mean.vi"("X"=w848) -> ("mean"=w847:dbl)  [unwired: 1 out]
        "Immersion Lens I read" <- w847
        n356 = call-poly <vilib>:"Mean.vi"("X"=w849) -> ("mean"=w851:dbl)  [unwired: 1 out]
        "Immersion Lens V read" <- w851
        n357 = call-poly <vilib>:"Mean.vi"("X"=w859) -> ("mean"=w855:dbl)  [unwired: 1 out]
        "Cathode I read" <- w855
        n358 = call-poly <vilib>:"Mean.vi"("X"=w858) -> ("mean"=w854:dbl)  [unwired: 1 out]
        "Cathode V read" <- w854
        n359 = call-poly <vilib>:"Mean.vi"("X"=w857) -> ("mean"=w853:dbl)  [unwired: 1 out]
        "Extractor V read" <- w853
        n360 = call-poly <vilib>:"Mean.vi"("X"=w856) -> ("mean"=w852:dbl)  [unwired: 1 out]
        "Extractor I read" <- w852
        n361 = shared-variable "SCA-cRIO\\global SCA shared var lib.lvlib\\Immersion Lens I read"(w847) -> ()  [unwired: 1 in, 1 out]
        n362 = shared-variable "SCA-cRIO\\global SCA shared var lib.lvlib\\Immersion Lens V read"(w851) -> ()  [unwired: 1 in, 1 out]
        n363 = shared-variable "SCA-cRIO\\global SCA shared var lib.lvlib\\Cathode I read"(w855) -> ()  [unwired: 1 in, 1 out]
        n364 = shared-variable "SCA-cRIO\\global SCA shared var lib.lvlib\\Cathode V read"(w854) -> ()  [unwired: 1 in, 1 out]
        n365 = shared-variable "SCA-cRIO\\global SCA shared var lib.lvlib\\Extractor V read"(w853) -> ()  [unwired: 1 in, 1 out]
        n366 = shared-variable "SCA-cRIO\\global SCA shared var lib.lvlib\\Extractor I read"(w852) -> ()  [unwired: 1 in, 1 out]
      }
    }
  }
  n367 = while {
    stop <- FALSE stop-if-true
    n368 = shared-variable "SCA-cRIO\\global SCA shared var lib.lvlib\\Bypass Control"() -> (w868:T1)  [unwired: 1 in, 1 out]
    "Bypass Control" <- w868
    n369 = Unbundle By Name(w868) -> ("Wheel GV Bypass"=w865:bool, "Sample Rod Bypass"=w864:bool, "Retract Rod Bypass"=w863:bool, "Insert Rod Bypass"=w862:bool)
    n370 = Or(x="Wheel GV Bypass", y=w865) -> (x .or. y?=w872:bool)
    n371 = Or(x="Sample Rod Bypass", y=w864) -> (x .or. y?=w871:bool)
    n372 = Or(x=w863, y="Retract Rod Bypass") -> (x .or. y?=w869:bool)
    n373 = Or(x=w862, y="Insert Rod Bypass") -> (x .or. y?=w870:bool)
    n374 = shared-variable ".\\local SCA shared var lib.lvlib\\Wheel GV Bypass"(w872) -> ()  [unwired: 1 in, 1 out]
    n375 = shared-variable ".\\local SCA shared var lib.lvlib\\Sample Rod Bypass"(w871) -> ()  [unwired: 1 in, 1 out]
    n376 = shared-variable ".\\local SCA shared var lib.lvlib\\Retract Rod Bypass"(w869) -> ()  [unwired: 1 in, 1 out]
    n377 = shared-variable ".\\local SCA shared var lib.lvlib\\Insert Rod Bypass"(w870) -> ()  [unwired: 1 in, 1 out]
  }
  n378 = timed-loop {
    timing: w6 -> [_]
    timing-out: [_] -> w5
    stop <- FALSE stop-if-true
    # "Encoder readback loop"
    n379 = node-c288() -> ()  [unwired: 1 in, 1 out]
    n380 = shared-variable "SCA-cRIO\\Mod6\\DIO0"() -> (w907:bool, error out=w890:errorcluster)  [unwired: 1 in]
    n381 = shared-variable "SCA-cRIO\\Mod6\\DIO1"(error in=w890) -> (w906:bool, error out=w889:errorcluster)
    n382 = shared-variable "SCA-cRIO\\Mod6\\DIO2"(error in=w889) -> (w897:bool, error out=w888:errorcluster)
    n383 = shared-variable "SCA-cRIO\\Mod6\\DIO3"(error in=w888) -> (w896:bool, error out=w887:errorcluster)
    n384 = shared-variable "SCA-cRIO\\Mod6\\DIO4"(error in=w887) -> (w905:bool, error out=w886:errorcluster)
    n385 = shared-variable "SCA-cRIO\\Mod6\\DIO5"(error in=w886) -> (w904:bool, error out=w885:errorcluster)
    n386 = shared-variable "SCA-cRIO\\Mod6\\DIO6"(error in=w885) -> (w903:bool, error out=w884:errorcluster)
    n387 = shared-variable "SCA-cRIO\\Mod6\\DIO7"(error in=w884) -> (w883:bool, error out=w882:errorcluster)
    n388 = shared-variable "SCA-cRIO\\Mod6\\DIO8"(error in=w882) -> (w902:bool, error out=w881:errorcluster)
    n389 = shared-variable "SCA-cRIO\\Mod6\\DIO9"(error in=w881) -> (w895:bool, error out=w880:errorcluster)
    n390 = shared-variable "SCA-cRIO\\Mod6\\DIO10"(error in=w880) -> (w901:bool, error out=w879:errorcluster)
    n391 = shared-variable "SCA-cRIO\\Mod6\\DIO11"(error in=w879) -> (w900:bool, error out=w878:errorcluster)
    n392 = shared-variable "SCA-cRIO\\Mod6\\DIO12"(error in=w878) -> (w899:bool, error out=w877:errorcluster)
    n393 = shared-variable "SCA-cRIO\\Mod6\\DIO13"(error in=w877) -> (w898:bool, error out=w876:errorcluster)
    n394 = Bundle By Name(cluster=T15 {"MSB"=FALSE, "13th bit"=FALSE, "12th bit"=FALSE, "11th bit"=FALSE, "10th bit"=FALSE, "9th bit"=FALSE, "8th bit"=FALSE, "7th bit"=FALSE, "6th bit"=FALSE, "5th bit"=FALSE, "4th bit"=FALSE, "3rd bit"=FALSE, "2nd bit"=FALSE, "LSB"=FALSE} ("Cluster"), "MSB"=w907, "13th bit"=w906, "12th bit"=w897, "11th bit"=w896, "10th bit"=w905, "9th bit"=w904, "8th bit"=w903, "7th bit"=w883, "6th bit"=w902, "5th bit"=w895, "4th bit"=w901, "3rd bit"=w900, "2nd bit"=w899, "LSB"=w898) -> (w909:T15)
    n395 = call "Encoder-Decoder.vi"("Encoder data"=w909) -> ("Raw bits"=→"Raw bits":bool[], "Converted bits"=→"Converted bits":bool[], "Encoder position"=w894:u16)  [unwired: 8 in]
    "Encoder position" <- w894
    n396 = shared-variable "SCA-cRIO\\global SCA shared var lib.lvlib\\Encoder position"(w894, error in=w876) -> (error out=w875:errorcluster)
    "Encoder loop error" <- w875
    n397 = shared-variable ".\\local SCA shared var lib.lvlib\\Encoder loop error"(w875) -> ()  [unwired: 1 in, 1 out]
    n398 = node-c288() -> ()  [unwired: 1 in, 1 out]
  }
  n399 = node-c288(w5) -> ()  [unwired: 1 out]
